vi "SpectrometerSpinCoater_v09.vi"() -> ()   [LabVIEW 2018]
uses:
  <instrlib>/Classes/CCD/Abstract_CCD/Abstract_CCD.lvclass
  <instrlib>/Classes/SpinCoater/SpinCoater.lvclass
  TypDef/DeviceQueue_TypeDef.ctl
  TypDef/DeviceQueue_Action.ctl
  TypDef/TabControl.ctl
  TypDef/DataQueue_TypeDef.ctl
  TypDef/DataQueue_Action.ctl
  <vilib>/Utility/error.llb/DialogType.ctl
  <instrlib>/Classes/CCD/Avantes/Avantes.lvclass
  C:/Program Files/National Instruments/LabVIEW 2018/instr.lib/Classes/CCD/Abstract_CCD/Abstract_CCD.lvclass
  <vilib>/Analysis/baseanly.llb/A x Vector.vi
  <vilib>/Analysis/NI_AALBase.lvlib
panel:
  out "Nr After Spin":u16
  out "Action":string="TimeOut"
  out "Time.spin":refnum<file>
  out "Meas.spin":refnum<file>
  out "Arduino":bool
  out "NKT":bool
  out "Spectromter":bool
  in  "Abort Button":bool
  in  "Stop Button":bool=TRUE
  in  "Tab Control":T1(tab)=enum."Settings"
  in  "Spin at end":bool
  in  "Duration after":dbl[unit]
  in  "periodic time":dbl[unit]
  in  "Program Spin Coater":T2(array[cluster])=[{"Speed (rpm)"=800.0, "Time (s)"=120.0, "Acc (rpm/s)"=0.0}]
  in  "Spectra Count":u16
  in  "Measure_MeasureSpectrum":bool
  out "Overall Time":dbl=121.5
  in  "Seconds after Spin":dbl[unit]=0.5
  in  "Seconds to Spin":dbl[unit]=1.0
  in  "Calculate Frames":bool=TRUE
  in  "Frames":i32=319737
  in  "StartMeasurement_Button":bool
  in  "Measure_Preview":bool
  out "Measure_Graph":T3(graph) caption="XY Graph"
  in  "Measure_FramesSpectrometer":dbl=200.0 caption="Frames for Spectrometer"
  in  "StartSpin_Button":bool
  in  "Record RefSpec":bool
  in  "Measure:\nRecord_Darkspec":bool
  in  "Measure_Comments":string="TL,  60°C, Blend P3HT 30g/L Verhältnis 1:1,2 PC70BM 24 g/L\nAuftrag während dem Spin\n" caption="Comments"
  in  "Measure_FileName":string="190624_JZ_P3HTPC70BM_TL_G17" caption="File Name"
  in  "Measure_SavePath":path=path "C:/Users/Cerberus/Desktop/Measurements" caption="Save Path"
  out "Measure_FrameRate":dbl[unit]=2631.5791015625 caption="Frame Rate"
  in  "Measure_IntegrationTime":dbl[unit]=3e-05 caption="Integration Time"
  out "SS_StepsLeft":dbl
  out "SS_TimePrediction":dbl[unit]
  out "Horizontal Progress Bar":u8(slide) scale=0.0..100.0
  in  "SpectralStability:\nRecord_Darkspec":bool
  in  "SpectralStability_Record":bool
  in  "SpectralStability_\nMeasurementNumber":u32 caption="Measurement Number"
  in  "SpectralStability_Duration":dbl[unit] caption="Duration"
  in  "Duration/Times":bool
  in  "SpectralStability_\nPeriodicTime":dbl[unit] caption="Periodic Time"
  in  "SpectralStability_MeasureSpectrum":bool
  in  "SpectralStability_Preview":bool
  out "SpectralStability_Graph":T3(graph) caption="XY Graph"
  in  "SpectralStability_FramesSpectrometer":dbl=200.0 caption="Frames for Spectrometer"
  in  "SpectralStability_Comments":string="Just for testing" caption="Comments"
  in  "SpectralStability_FileName":string="TestingAfter" caption="File Name"
  in  "SpectralStability_SavePath":path=path "C:/Users/Timo/Desktop/Test/180824" caption="Save Path"
  out "SpectralStability_FrameRate":dbl[unit]=2631.5791015625 caption="Frame Rate"
  in  "SpectralStability_IntegrationTime":dbl[unit]=3e-05 caption="Integration Time"
  in  "Dividider Get Spectra":u32=1 min=1
  in  "Automatically \nadjust count":bool=TRUE
  in  "Reset Count\nafter Spin Coating":bool=TRUE
  in  "Speed":dbl
  in  "Milliseconds":dbl
  in  "Debug":bool
  in  "Port Arduino":refnum<visa-resource-name>="COM7"
  out "Error Arduino":bool caption="Error"
  in  "Init_Arduino":bool caption="Init"
  out "Caption_Settings_Arduino":string="Arduino"
  out "Caption_Settings_NKT":string="NKT Laser"
  out "Error_Spectromter":bool caption="Error"
  in  "Init_Spectrometer":bool caption="Init"
  out "Caption_Settings_Spectrometer":string="Spectromter"
  # "Speed (rpm)   Time (s)        Acceleration \n                                               (rpm/s)"
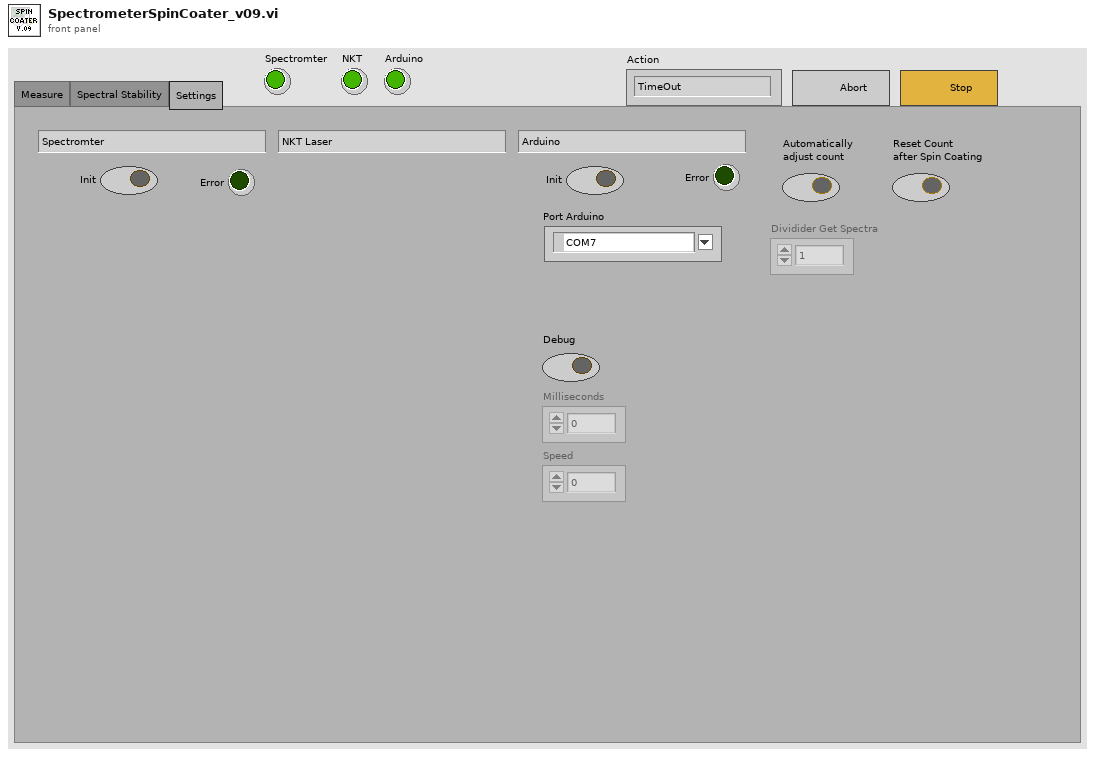
[diagram p1: front panel]
types:
  T1 = enum32{"Measure", "Spectral Stability", "Settings"}
  T2 = cluster{"Speed (rpm)":dbl, "Time (s)":dbl, "Acc (rpm/s)":dbl}[]
  T3 = cluster{"Wavlength":dbl[unit][], "Image":dbl[]}[]
  T4 = cluster{"Dark":cluster{"Image":dbl[][][], "Frame Size":cluster{"F":i32, "Y":i32, "X":i32}}[], "Ref":cluster{"Image":dbl[][][], "Frame Size":cluster{"F":i32, "Y":i32, "X":i32}}[], "Wavlength":dbl[unit][], "spec":dbl[][]}
  T5 = cluster{"Abstract_CCD.lvclass":refnum<class "Abstract_CCD.lvclass">, "SpinCoater.lvclass":refnum<class "SpinCoater.lvclass">}
  T6 = typedef "DataQueue_TypeDef.ctl" = cluster{"QueueAction":T7, "Data":cluster{"Image":dbl[][][], "Frame Size":cluster{"F":i32, "Y":i32, "X":i32}}[], "Data_Raw":cluster{"Image":dbl[][][], "Frame Size":cluster{"F":i32, "Y":i32, "X":i32}}[], "Data_Dark":cluster{"Image":dbl[][][], "Frame Size":cluster{"F":i32, "Y":i32, "X":i32}}[], "Data_Ref":cluster{"Image":dbl[][][], "Frame Size":cluster{"F":i32, "Y":i32, "X":i32}}[], "Device Information":string[], "Numeric Control":dbl, "Boolean":bool, "Wavelength":dbl[unit][], "Time":dbl[], "Time Stamp":timestamp, "Numeric Control 2":dbl, "TabControl":T8}
  T7 = typedef "DataQueue_Action.ctl" = enum16{"TimeOut", "Close_Program", "Abort", "Stop_Measurement", "Measure_InSituSpinCoating", "Measure_Spectrum", "Measure_SpectrumAdvanced", "Measure_SpectralStability", "Save_InSitu", "Save_SpectralStability", "Set_Ref", "Set_Dark", "Set_Wavelength", "Spectrometer_Measure", "Spectrometer_Preview", "Transfer_Settings"}
  T8 = typedef "TabControl.ctl" = enum16{"Measure", "Spectral Stability", "Settings"}
  T9 = typedef "DeviceQueue_TypeDef.ctl" = cluster{"QueueAction":T10, "Numeric 1":dbl, "Numeric 2":dbl, "Boolean 1":bool, "Boolean 2":bool, "Spin Program":dbl[][], "Spin Prg v07":cluster{"Speed (rpm)":dbl, "Time (s)":dbl, "Acc (rpm/s)":dbl}[], "Time Stamp":timestamp, "TabControl":T8}
  T10 = typedef "DeviceQueue_Action.ctl" = enum16{"TimeOut", "Wait", "Close_Program", "Abort", "Spectrometer_Init", "Spectrometer_Close", "Spectrometer_DeviceInformation", "Spectrometer_Measure", "Spectrometer_MeasureAdvanced", "Spectrometer_Preview", "Spectrometer_Abort", "Spectrometer_StartMeasurement", "Spectrometer_GetData", "Spectrometer_StopMeasurement", "Spectrometer_SetIntegrationTime", "Spectrometer_SetFrames", "Spectrometer_SetDarkspec", "Spectrometer_SetReference", "Spectrometer_SetTriggerMode", "Laser_Init", "Laser_Close", "Arduino_Init", "Arduino_Close", "Arduino_LoadProgram", "Arduino_StartProgram", "Arduino_SetSpeed", "Arduino_SetMillis", "Arduino_StopSpin", "Measure_InSitu", "Measure_Spectrum", "Measure_InSituAdvanced", "Measure_SpectralStability", "Measure_Stop"}
  T11 = cluster{"Image":dbl[][][], "Frame Size":cluster{"F":i32, "Y":i32, "X":i32}}[]
  T12 = typedef "DialogType.ctl" = u16
  T13 = enum16{"open", "replace", "create", "open or create", "replace or create", "replace or create with confirmation"}
  T14 = cluster{"Image":dbl[][][], "Frame Size":cluster{"F":i32, "Y":i32, "X":i32}}
  T15 = cluster{"Wavlength":dbl[unit][], "A x Vector":dbl[]}
  T16 = cluster{"Wavlength":dbl[unit][], "A x Vector":dbl[]}[]
  T17 = cluster{u16[][][], u16[][][], dbl[], "Numeric Control":dbl, "Numeric Control 2":dbl}
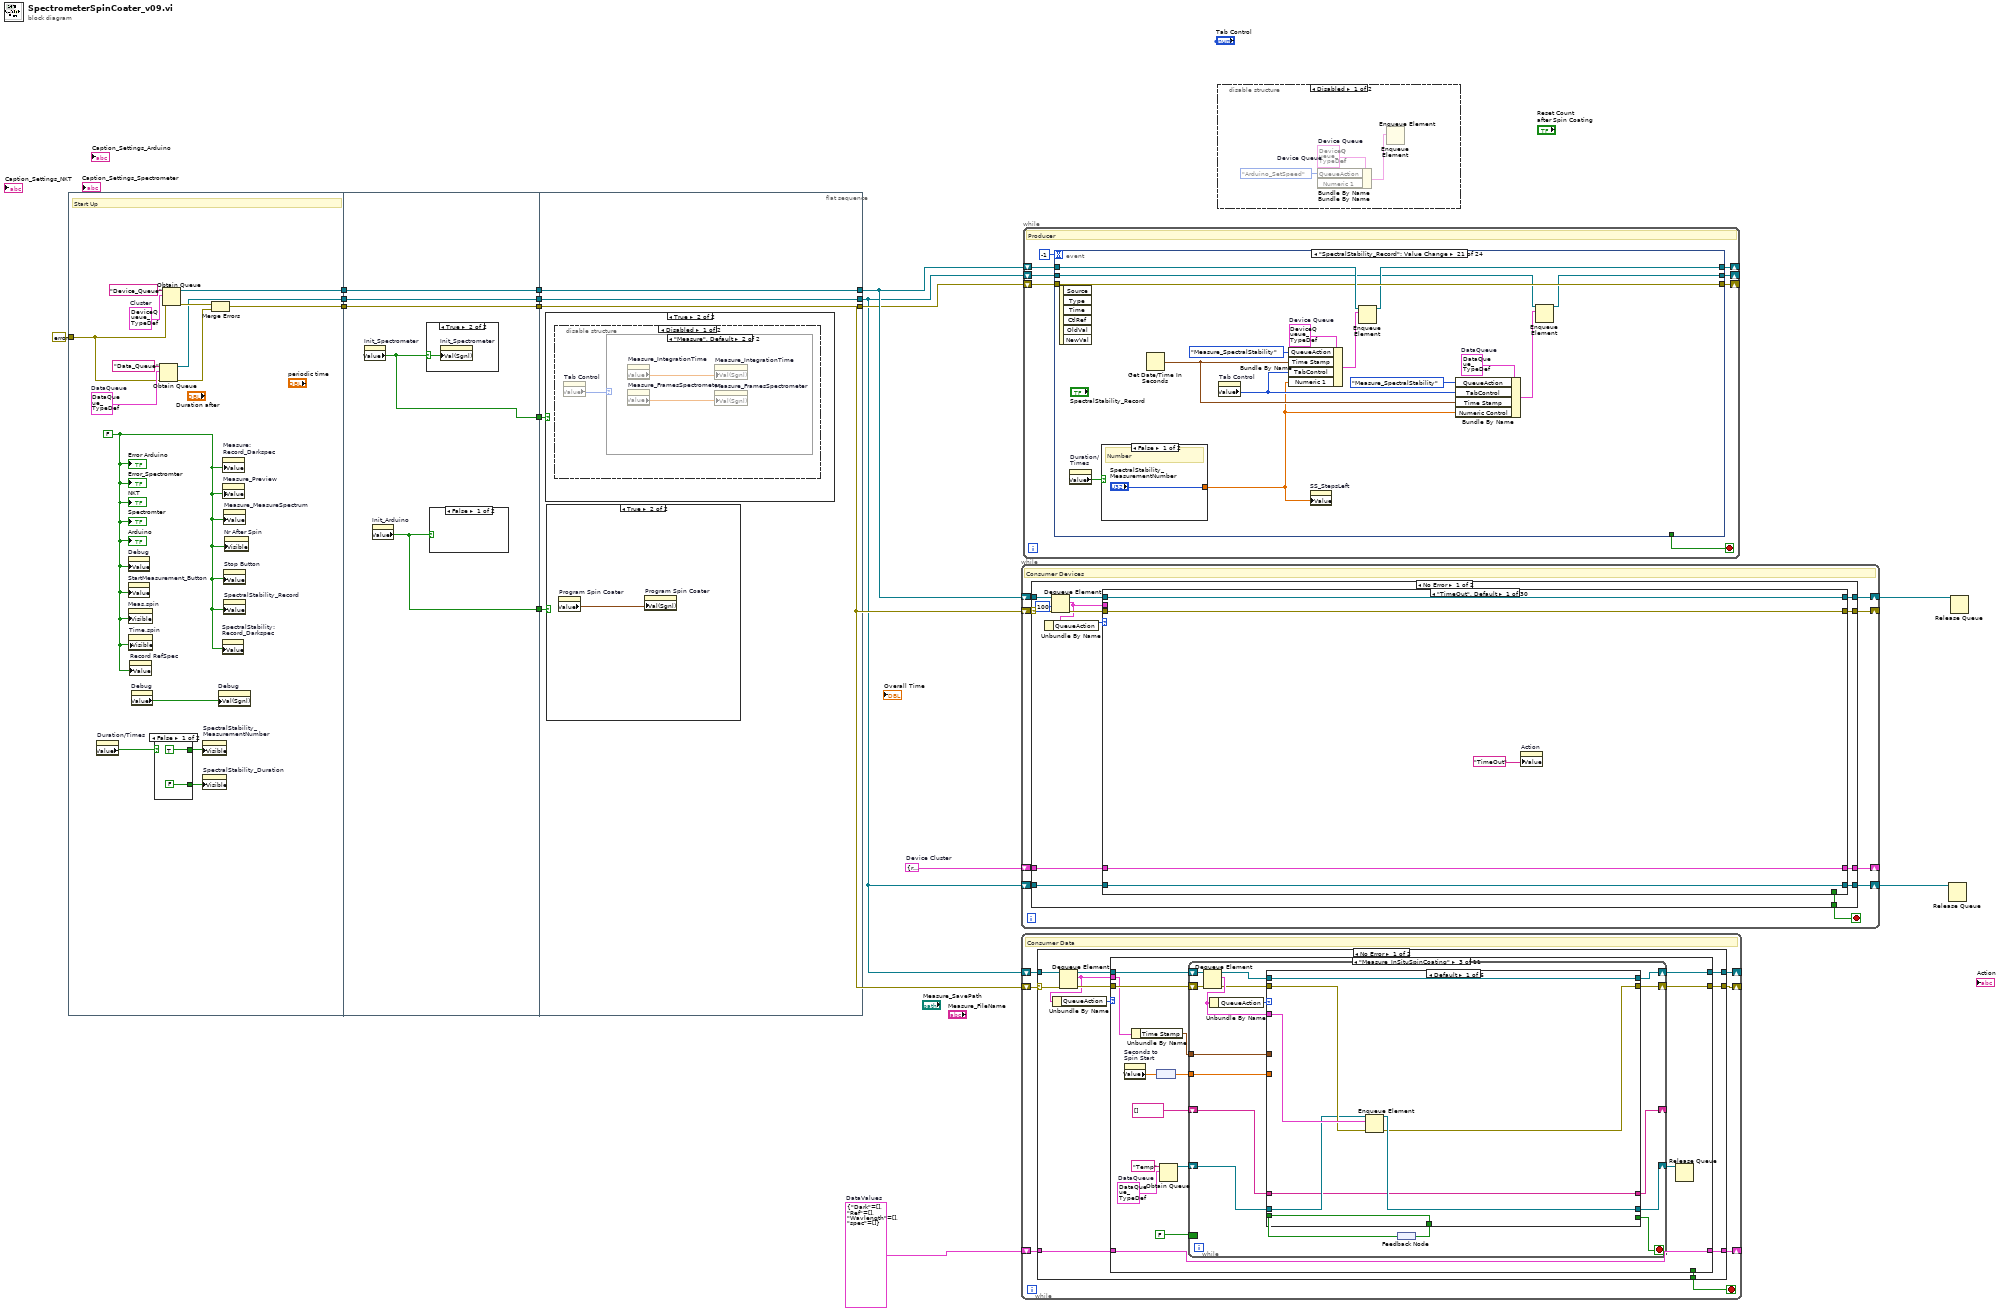
[diagram p0: block diagram]
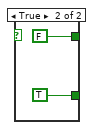
[diagram p3: hidden frame]
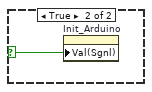
[diagram p4: hidden frame]
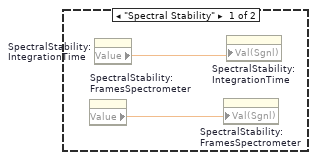
[diagram p8: hidden frame]
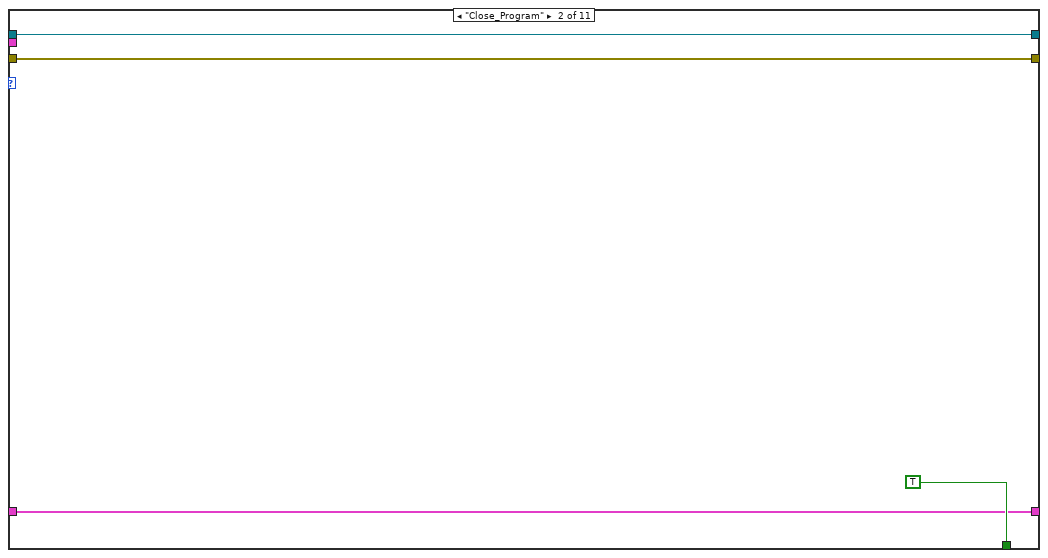
[diagram p11: hidden frame]
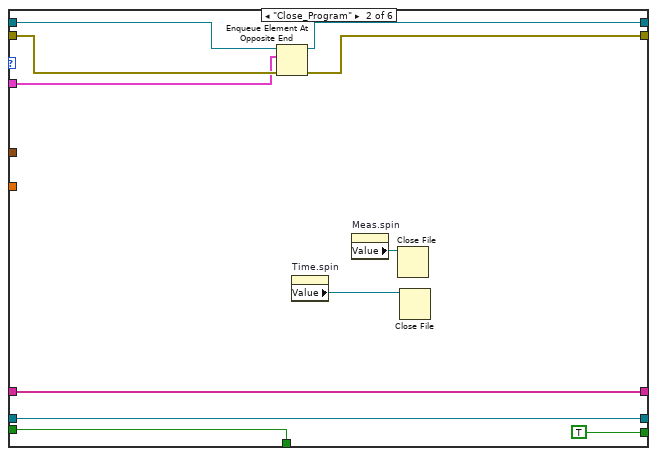
[diagram p12: hidden frame]
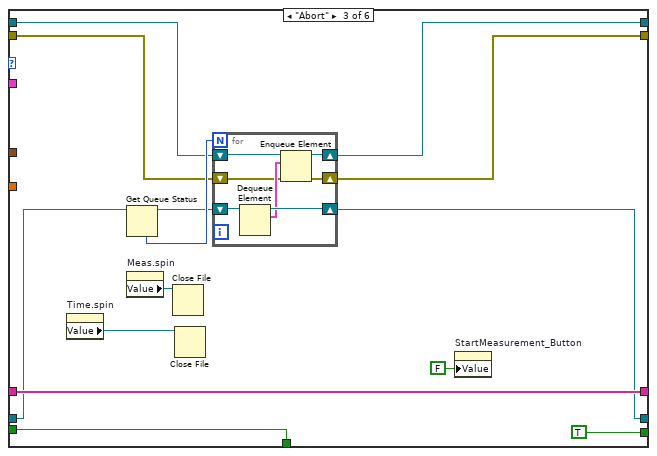
[diagram p13: hidden frame]
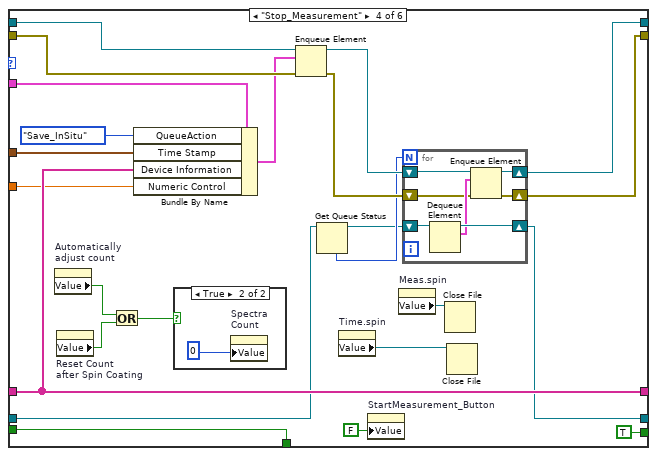
[diagram p14: hidden frame]
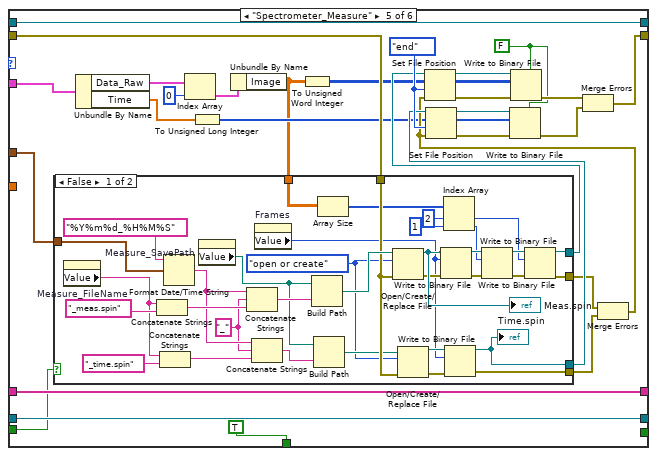
[diagram p16: hidden frame]
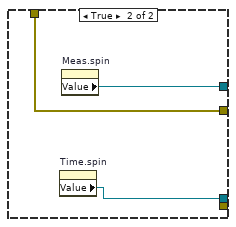
[diagram p17: hidden frame]
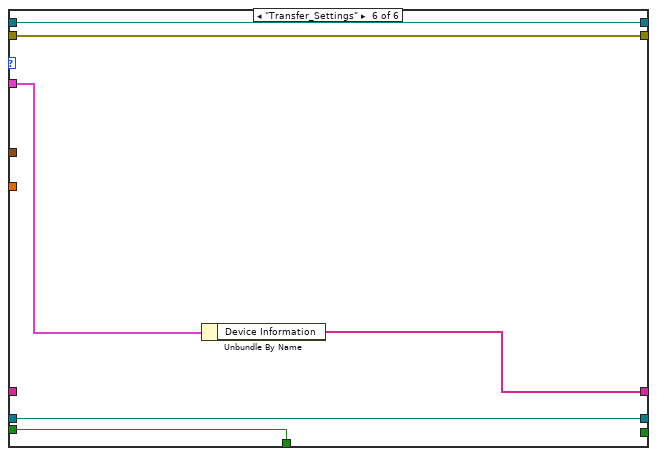
[diagram p18: hidden frame]
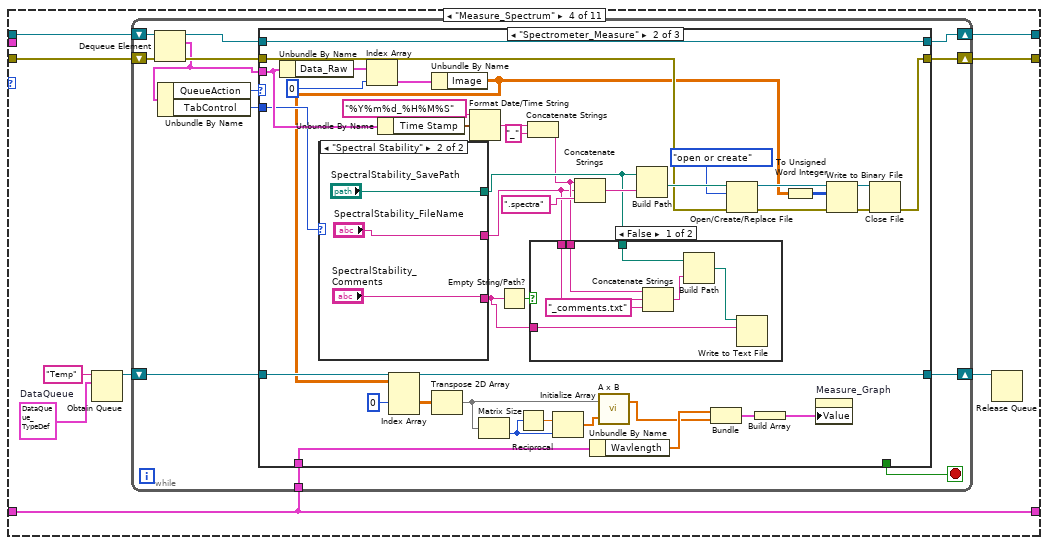
[diagram p19: hidden frame]
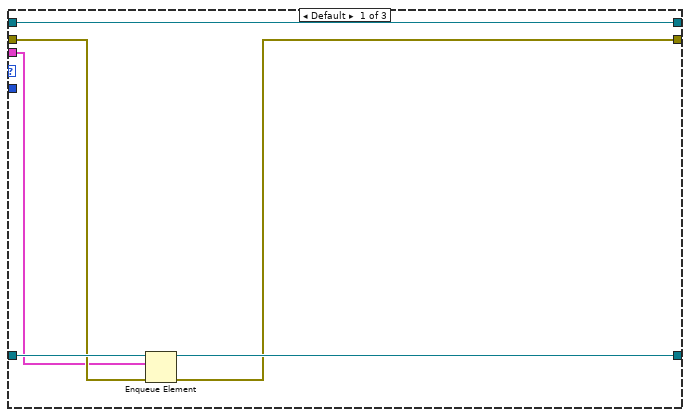
[diagram p20: hidden frame]
diagram:
  w6 = T4 {"Dark"=[], "Ref"=[], "Wavlength"=[], "spec"=[]}  # DataValues
  w11 = T5 {"Abstract_CCD.lvclass"=refnum, "SpinCoater.lvclass"=refnum}  # Device Cluster
  n1 = flat-sequence {
    tunnel: errorcluster {"status"=FALSE, "code"=0, "source"=""} ("error constant") -> [w26]
    tunnel: [w29] -> w15
    tunnel: [w23] -> w14
    tunnel: [w22] -> w13
    tunnel: w15 -> [w40]
    tunnel: w14 -> [w39]
    tunnel: w13 -> [w38]
    tunnel: [w40] -> w5
    tunnel: [w39] -> w4
    tunnel: [w38] -> w3
    tunnel: [w37] -> w2
    tunnel: [w36] -> w1
    tunnel: [w45] -> w8
    tunnel: [w46] -> w7
    tunnel: [w47] -> w12
    tunnel: w5 -> [w47]
    tunnel: w4 -> [w46]
    tunnel: w3 -> [w45]
    tunnel: w2 -> [w44]
    tunnel: w1 -> [w43]
    frame #0 {
      w27 = T6 {"QueueAction"=enum."TimeOut", "Data"=[], "Data_Raw"=[], "Data_Dark"=[], "Data_Ref"=[], "Device Information"=[], "Numeric Control"=0.0, "Boolean"=FALSE, "Wavelength"=[], "Time"=[], "Time Stamp"=timestamp(0 s since 1904-01-01), "Numeric Control 2"=0.0, "TabControl"=enum."Measure"}  # DataQueue
      w30 = T9 {"QueueAction"=enum."TimeOut", "Numeric 1"=0.0, "Numeric 2"=0.0, "Boolean 1"=FALSE, "Boolean 2"=FALSE, "Spin Program"=[], "Spin Prg v07"=[], "Time Stamp"=timestamp(0 s since 1904-01-01), "TabControl"=enum."Measure"}  # Cluster
      w17 = FALSE ("Error Arduino")
      # "Start Up"
      n2 = property on="Duration/Times" class="Bool (strict)"() -> ("Value"=w18:bool)  [unwired: 2 in, 2 out]
      n3 = property on="Debug" class="Bool (strict)"("Value"=w17) -> ()  [unwired: 2 in, 2 out]
      n4 = property on="StartMeasurement_Button" class="Bool (strict)"("Value"=w17) -> ()  [unwired: 2 in, 2 out]
      n5 = property on="Meas.spin" class="Ref (strict)"("Visible"=w17) -> ()  [unwired: 2 in, 2 out]
      n6 = property on="Time.spin" class="Ref (strict)"("Visible"=w17) -> ()  [unwired: 2 in, 2 out]
      n7 = property on="Record RefSpec" class="Bool (strict)"("Value"=w17) -> ()  [unwired: 2 in, 2 out]
      n8 = property on="Debug" class="Bool (strict)"() -> ("Value"=w21:bool)  [unwired: 2 in, 2 out]
      n9 = case shown="False" w18 {
        tunnel: [FALSE TRUE] -> w20
        tunnel: [TRUE FALSE] -> w19
        frame False {
        }
        frame True {
        }
      }
      n10 = Obtain Queue(name (unnamed)="Data_Queue", element data type=w27, error in (no error)=w26) -> (queue out=w23:refnum<queue>, error out=w24:errorcluster)  [unwired: 2 in, 1 out]
      n11 = Obtain Queue(name (unnamed)="Device_Queue", element data type=w30, error in (no error)=w26) -> (queue out=w29:refnum<queue>, error out=w25:errorcluster)  [unwired: 2 in, 1 out]
      n12 = property on="SpectralStability_\nMeasurementNumber" class="DigNum (strict)"("Visible"=w19) -> ()  [unwired: 2 in, 2 out]
      n13 = property on="SpectralStability_Duration" class="DigNum (strict)"("Visible"=w20) -> ()  [unwired: 2 in, 2 out]
      n14 = Merge Errors(w25, w24) -> (w22:errorcluster)
      n15 = property on="Debug" class="Bool (strict)"("Val(Sgnl)"=w21) -> ()  [unwired: 2 in, 2 out]
      n16 = property on="SpectralStability:\nRecord_Darkspec" class="Bool (strict)"("Value"=w17) -> ()  [unwired: 2 in, 2 out]
      n17 = property on="Measure:\nRecord_Darkspec" class="Bool (strict)"("Value"=w17) -> ()  [unwired: 2 in, 2 out]
      n18 = property on="Measure_Preview" class="Bool (strict)"("Value"=w17) -> ()  [unwired: 2 in, 2 out]
      n19 = property on="Measure_MeasureSpectrum" class="Bool (strict)"("Value"=w17) -> ()  [unwired: 2 in, 2 out]
      n20 = property on="Stop Button" class="Bool (strict)"("Value"=w17) -> ()  [unwired: 2 in, 2 out]
      n21 = property on="SpectralStability_Record" class="Bool (strict)"("Value"=w17) -> ()  [unwired: 2 in, 2 out]
      n22 = property on="Nr After Spin" class="DigNum (strict)"("Visible"=w17) -> ()  [unwired: 2 in, 2 out]
      "Error_Spectromter" <- w17
      "Error Arduino" <- w17
      "Spectromter" <- w17
      "NKT" <- w17
      "Arduino" <- w17
    }
    frame #1 {
      n23 = property on="Init_Spectrometer" class="Bool (strict)"() -> ("Value"=w37:bool)  [unwired: 2 in, 2 out]
      n24 = property on="Init_Arduino" class="Bool (strict)"() -> ("Value"=w36:bool)  [unwired: 2 in, 2 out]
      n25 = case shown="True" w37 {
        selector: w37 -> [_ w42]
        frame False {
        }
        frame True {
          n26 = property on="Init_Spectrometer" class="Bool (strict)"("Val(Sgnl)"=w42) -> ()  [unwired: 2 in, 2 out]
        }
      }
      n27 = case shown="False" w36 {
        selector: w36 -> [_ w41]
        frame False {
        }
        frame True {
          n28 = property on="Init_Arduino" class="Bool (strict)"("Val(Sgnl)"=w41) -> ()  [unwired: 2 in, 2 out]
        }
      }
    }
    frame #2 {
      n29 = case shown="True" w44 {
        frame False {
        }
        frame True {
          n30 = disable-structure shown="Disabled" {
            frame Disabled {
              n31 = property on="Tab Control" class="TabCtl (strict)"() -> ("Value"=w49:T1)  [unwired: 2 in, 2 out]
              n32 = case shown="\"Measure\", Default" w49 {
                frame "Spectral Stability" {
                  n33 = property on="SpectralStability:\nFramesSpectrometer" class="DigNum (strict)"() -> ("Value"=w50:dbl)  [unwired: 2 in, 2 out]
                  n34 = property on="SpectralStability:\nIntegrationTime" class="DigNum (strict)"() -> ("Value"=w51:dbl[unit])  [unwired: 2 in, 2 out]
                  n35 = property on="SpectralStability:\nFramesSpectrometer" class="DigNum (strict)"("Val(Sgnl)"=w50) -> ()  [unwired: 2 in, 2 out]
                  n36 = property on="SpectralStability:\nIntegrationTime" class="DigNum (strict)"("Val(Sgnl)"=w51) -> ()  [unwired: 2 in, 2 out]
                }
                frame "Measure", Default {
                  n37 = property on="Measure_IntegrationTime" class="DigNum (strict)"() -> ("Value"=w52:dbl[unit])  [unwired: 2 in, 2 out]
                  n38 = property on="Measure_FramesSpectrometer" class="DigNum (strict)"() -> ("Value"=w53:dbl)  [unwired: 2 in, 2 out]
                  n39 = property on="Measure_IntegrationTime" class="DigNum (strict)"("Val(Sgnl)"=w52) -> ()  [unwired: 2 in, 2 out]
                  n40 = property on="Measure_FramesSpectrometer" class="DigNum (strict)"("Val(Sgnl)"=w53) -> ()  [unwired: 2 in, 2 out]
                }
              }
            }
            frame Enabled {
            }
          }
        }
      }
      n41 = case shown="True" w43 {
        frame False {
        }
        frame True {
          n42 = property on="Program Spin Coater" class="Arr (strict)"() -> ("Value"=w48:T2)  [unwired: 2 in, 2 out]
          n43 = property on="Program Spin Coater" class="Arr (strict)"("Val(Sgnl)"=w48) -> ()  [unwired: 2 in, 2 out]
        }
      }
    }
  }
  n44 = while {
    shift-right: [w58] -> _
    shift-left: w8 -> [w62]
    shift-right: [w59] -> w10
    shift-left: w12 -> [w61]
    shift-right: [w56] -> w9
    shift-left: w7 -> [w57]
    shift-right: [w54] -> _
    shift-left: w11 -> [w55]
    stop <- w60 stop-if-true
    # "Consumer Devices"
    n45 = case shown="No Error" w62 {
      selector: w62 -> [w75 w763]
      tunnel: w61 -> [w76 w764]
      tunnel: [w72 _] -> w60
      tunnel: [w71 w764] -> w59
      tunnel: [w69 w760] -> w58
      tunnel: w57 -> [w67 w758]
      tunnel: [w68 w758] -> w56
      tunnel: w55 -> [w66 w759]
      tunnel: [w65 w759] -> w54
      frame No Error {
        n46 = Dequeue Element(queue=w76, timeout in ms (-1)=100, error in (no error)=w75) -> (queue out=w74:refnum<queue>, element=w64:T9, error out=w70:errorcluster)  [unwired: 1 out]
        n47 = Unbundle By Name(w64) -> ("QueueAction"=w73:T10)
        n48 = case shown="\"TimeOut\", Default" w73 {
          tunnel: w74 -> [w81 w102 w143 w161 w172 w227 w246 w271 w282 w305 w312 w331 w333 w364 w383 w398 w408 w420 w432 w453 w475 w480 w487 w499 w505 w515 w561 w651 w719 w729]
          tunnel: [_ _ w145 _ _ _ _ _ _ _ _ _ _ _ _ _ _ _ _ _ _ _ _ _ _ _ _ _ _ _] -> w72
          tunnel: [w81 w102 w128 w147 w168 w227 w246 w271 w283 w305 w312 w331 w333 w364 w383 w398 w408 w420 w431 w453 w475 w480 w487 w499 w505 w515 w523 w577 w710 w732] -> w71
          tunnel: w70 -> [w80 w101 w127 w160 w183 w228 w245 w270 w278 w308 w316 w328 w343 w362 w373 w389 w405 w416 w427 w456 w469 w477 w485 w494 w502 w508 w517 w612 w718 w728]
          tunnel: [w80 w101 w126 w148 w171 w222 w244 w269 w276 w306 w313 w318 w337 w361 w368 w385 w403 w410 w430 w455 w466 w476 w483 w493 w501 w507 w524 w578 w709 w733] -> w69
          tunnel: [w78 w99 w125 w165 w169 w224 w237 w251 w287 w304 w311 w322 w345 w365 w377 w392 w399 w412 w434 w454 w474 w482 w491 w497 w506 w510 w532 w624 w717 w749] -> w68
          tunnel: w67 -> [w78 w99 w125 w165 w170 w224 w236 w260 w288 w304 w311 w323 w345 w365 w380 w395 w399 w414 w434 w454 w474 w482 w491 w497 w506 w511 w532 w624 w717 w749]
          tunnel: w66 -> [w79 w100 w124 w164 w180 w226 w243 w268 w281 w303 w315 w324 w336 w358 w376 w391 w402 w409 w429 w449 w468 w481 w490 w496 w504 w509 w564 w654 w716 w748]
          tunnel: [w79 w100 w124 w164 w174 w225 w243 w268 w280 w301 w310 w324 w334 w359 w375 w390 w400 w409 w433 w447 w465 w481 w490 w496 w504 w509 w564 w654 w716 w748] -> w65
          tunnel: w64 -> [_ w95 _ _ w167 _ w235 w262 w274 _ _ w330 w340 w366 _ _ w406 _ _ _ w473 _ w489 w498 _ _ _ w594 w707 w723]
          frame "TimeOut", Default {
            n49 = property on="Action" class="Str"("Value"="TimeOut" ("Action")) -> ()  [unwired: 2 in, 2 out]
          }
          frame "Wait" {
            n50 = flat-sequence {
              tunnel: [w113] -> w96
              tunnel: w95 -> [w113]
              tunnel: [w112] -> w93
              frame #0 {
                n51 = Tick Count (ms)() -> (millisecond timer value=w112:u32)
              }
            }
            n52 = Unbundle By Name(w96) -> ("Numeric 1"=w87:dbl)
            n53 = property on="SS:PeriodicTime" class="DigNum (strict)"() -> ("Value"=w89:dbl[unit])  [unwired: 2 in, 2 out]
            n54 = Multiply(x=w87, y=1000.0) -> (x*y=w91:dbl)
            n55 = node(w87) -> (w88:dbl[unit])
            n56 = property on="SS_StepsLeft" class="DigNum (strict)"() -> ("Value"=w86:dbl)  [unwired: 2 in, 2 out]
            n57 = Round Toward -Infinity(1:w87) -> (0:w90:dbl)
            n58 = Subtract(x=w89, y=w88) -> (x-y=w83:dbl[unit])
            n59 = Decrement(x=w86) -> (x-1=w85:dbl)
            n60 = Multiply(x=w85, y=w89) -> (x*y=w84:dbl[unit])
            n61 = Add(x=w84, y=w83) -> (x+y=w82:dbl[unit])
            n62 = for {
              N: w90 -> [_]
              tunnel: 1000.0 ("y") -> [w114]
              tunnel: [w122] -> w94
              tunnel: w82 -> [w119]
              i -> [w117]
              stop <- w122 stop-if-true
              n63 = Increment(x=w117) -> (x+1=w115:i32)
              n64 = Multiply(x=w114, y=w115) -> (x*y=w116:dbl)
              n65 = node(w116) -> (w118:dbl[unit])
              n66 = property on="Stop Button" class="Bool (strict)"() -> ("Value"=w122:bool)  [unwired: 2 in, 2 out]
              n67 = Wait (ms)(milliseconds to wait=w114) -> (millisecond timer value=w120:u32)
              n68 = Subtract(x=w119, y=w118) -> (x-y=w121:dbl[unit])
              n69 = flat-sequence {
                tunnel: w121 -> [w123]
                tunnel: w120 -> [_]
                frame #0 {
                  n70 = property on="SS_TimePrediction" class="DigNum (strict)"("Value"=w123) -> ()  [unwired: 2 in, 2 out]
                }
              }
            }
            n71 = property on="Action" class="Str"("Value"="Wait" ("Action")) -> ()  [unwired: 2 in, 2 out]
            n72 = case shown="False" w94 {
              tunnel: w93 -> [w108 _]
              tunnel: w91 -> [w103 _]
              frame False {
                n73 = flat-sequence {
                  tunnel: [w111] -> w109
                  frame #0 {
                    n74 = Tick Count (ms)() -> (millisecond timer value=w111:u32)
                  }
                }
                n75 = Subtract(x=w109, y=w108) -> (x-y=w107:u32)
                n76 = To Double Precision Float(number=w107) -> (double precision float=w104:dbl)
                n77 = Subtract(x=w103, y=w104) -> (x-y=w105:dbl)
                n78 = Greater Than 0?(x=w105) -> (x > 0?=w106:bool)
                n79 = case shown="True" w106 {
                  tunnel: w105 -> [_ w110]
                  frame False {
                  }
                  frame True {
                    n80 = Wait (ms)(milliseconds to wait=w110) -> ()  [unwired: 1 out]
                  }
                }
              }
              frame True {
                # "If Aborted, do nothing"
              }
            }
          }
          frame "Close_Program" {
            w144 = T9 {"QueueAction"=enum."TimeOut", "Numeric 1"=0.0, "Numeric 2"=0.0, "Boolean 1"=FALSE, "Boolean 2"=FALSE, "Spin Program"=[], "Spin Prg v07"=[], "Time Stamp"=timestamp(0 s since 1904-01-01), "TabControl"=enum."Measure"}  # Device Queue
            n81 = Bundle By Name(cluster=w144, "QueueAction"=DeviceQueue_Action."Spectrometer_Close") -> (w139:T9)
            n82 = Bundle By Name(cluster=w139, "QueueAction"=DeviceQueue_Action."Laser_Close") -> (w137:T9)
            n83 = Bundle By Name(cluster=w137, "QueueAction"=DeviceQueue_Action."Arduino_Close") -> (w131:T9)
            n84 = Enqueue Element(queue=w143, element=w139, error in (no error)=w127) -> (queue out=w141:refnum<queue>, error out=w136:errorcluster)  [unwired: 1 in, 1 out]
            n85 = Bundle By Name(cluster=w131, "QueueAction"=DeviceQueue_Action."Close_Program") -> (w129:T9)
            n86 = Enqueue Element(queue=w141, element=w137, error in (no error)=w136) -> (queue out=w135:refnum<queue>, error out=w134:errorcluster)  [unwired: 1 in, 1 out]
            n87 = Enqueue Element(queue=w135, element=w131, error in (no error)=w134) -> (queue out=w133:refnum<queue>, error out=w132:errorcluster)  [unwired: 1 in, 1 out]
            n88 = Enqueue Element(queue=w133, element=w129, error in (no error)=w132) -> (queue out=w128:refnum<queue>, error out=w126:errorcluster)  [unwired: 1 in, 1 out]
            n89 = First Call?() -> (First Call?: T/F=w146:bool)
            n90 = Not(x=w146) -> (.not. x?=w145:bool)
          }
          frame "Abort" {
            w163 = T9 {"QueueAction"=enum."TimeOut", "Numeric 1"=0.0, "Numeric 2"=0.0, "Boolean 1"=FALSE, "Boolean 2"=FALSE, "Spin Program"=[], "Spin Prg v07"=[], "Time Stamp"=timestamp(0 s since 1904-01-01), "TabControl"=enum."Measure"}  # Device Queue
            n91 = Flush Queue(queue=w161, error in (no error)=w160) -> (queue out=w159:refnum<queue>, error out=w158:errorcluster)  [unwired: 1 out]
            n92 = Bundle By Name(cluster=w163, "QueueAction"=DeviceQueue_Action."Spectrometer_StopMeasurement") -> (w155:T9)
            n93 = Bundle By Name(cluster=w155, "QueueAction"=DeviceQueue_Action."Arduino_StopSpin") -> (w151:T9)
            n94 = Enqueue Element(queue=w159, element=w155, error in (no error)=w158) -> (queue out=w157:refnum<queue>, error out=w156:errorcluster)  [unwired: 1 in, 1 out]
            n95 = Bundle By Name(cluster=w151, "QueueAction"=DeviceQueue_Action."Measure_Stop") -> (w150:T9)
            n96 = Enqueue Element(queue=w157, element=w151, error in (no error)=w156) -> (queue out=w153:refnum<queue>, error out=w152:errorcluster)  [unwired: 1 in, 1 out]
            n97 = Enqueue Element(queue=w153, element=w150, error in (no error)=w152) -> (queue out=w147:refnum<queue>, error out=w148:errorcluster)  [unwired: 1 in, 1 out]
          }
          frame "Spectrometer_Init" {
            n98 = call-dynamic "Init.vi"("error in (no error)"=w183, "Variant"=0, "Avantes in"=refnum<class "Avantes.lvclass"> refnum ("Avantes.lvclass")) -> ("error out"=w182:errorcluster, "Avantes out"=w181:refnum<class "Avantes.lvclass">)  [unwired: 7 in]
            n99 = call-dynamic "IsInit.vi"("error in (no error)"=w182, "Avantes in"=w181) -> ("error out"=w178:errorcluster, "Is Init?"=w177:bool, "Avantes out"=w179:refnum<class "Avantes.lvclass">)  [unwired: 7 in]
            n100 = Unbundle By Name(w167) -> ("TabControl"=w166:T8)
            n101 = property on="Spectromter" class="Bool (strict)"("Value"=w177) -> ()  [unwired: 2 in, 2 out]
            n102 = property on="Init_Spectrometer" class="Bool (strict)"("Value"=w177) -> ()  [unwired: 2 in, 2 out]
            n103 = call-dynamic "Set_ExposurePerFrame.vi"("error in (no error)"=w178, "Exposure per Frame"=1, "Avantes in"=w179) -> ("error out"=w173:errorcluster, "Avantes out"=w176:refnum<class "Avantes.lvclass">)  [unwired: 7 in]
            n104 = case shown="False" w177 {
              tunnel: w176 -> [_ w206]
              tunnel: w173 -> [w189 w204]
              tunnel: [refnum<class "Abstract_CCD.lvclass"> refnum ("Abstract_CCD.lvclass") w205] -> w175
              tunnel: w172 -> [w187 w216]
              tunnel: [w189 w209] -> w171
              tunnel: w170 -> [w188 w201]
              tunnel: [w188 w199] -> w169
              tunnel: [w187 w197] -> w168
              tunnel: w167 -> [_ w194]
              tunnel: w166 -> [_ w193]
              frame False {
              }
              frame True {
                w207 = T6 {"QueueAction"=enum."TimeOut", "Data"=[], "Data_Raw"=[], "Data_Dark"=[], "Data_Ref"=[], "Device Information"=[], "Numeric Control"=0.0, "Boolean"=FALSE, "Wavelength"=[], "Time"=[], "Time Stamp"=timestamp(0 s since 1904-01-01), "Numeric Control 2"=0.0, "TabControl"=enum."Measure"}  # DataQueue
                n105 = case shown="\"Spectral Stability\"" w193 {
                  tunnel: [w218 w220] -> w192
                  tunnel: [w217 w219] -> w191
                  frame "Measure", Default {
                    n106 = property on="Measure_IntegrationTime" class="DigNum (strict)"() -> ("Value"=w218:dbl[unit])  [unwired: 2 in, 2 out]
                    n107 = property on="Measure_FramesSpectrometer" class="DigNum (strict)"() -> ("Value"=w217:dbl)  [unwired: 2 in, 2 out]
                  }
                  frame "Spectral Stability" {
                    n108 = property on="SpectralStability_FramesSpectrometer" class="DigNum (strict)"() -> ("Value"=w219:dbl)  [unwired: 2 in, 2 out]
                    n109 = property on="SpectralStability_IntegrationTime" class="DigNum (strict)"() -> ("Value"=w220:dbl[unit])  [unwired: 2 in, 2 out]
                  }
                }
                n110 = call-dynamic "Get_WavelengthAxis.vi"("error in (no error)"=w204, "Avantes in"=w206) -> ("error out"=w203:errorcluster, "lambda"=w198:dbl[unit][], "Avantes out"=w205:refnum<class "Avantes.lvclass">)  [unwired: 7 in]
                n111 = Unbundle(w203) -> ("status"=w202:bool)  [unwired: 2 out]
                n112 = property on="Error_Spectromter" class="Bool (strict)"("Value"=w202) -> ()  [unwired: 2 in, 2 out]
                n113 = property on="Calculate Frames" class="Bool (strict)"() -> ("Value"=w195:bool)  [unwired: 2 in, 2 out]
                n114 = Bundle By Name(cluster=w207, "QueueAction"=DataQueue_Action."Set_Wavelength", "Wavelength"=w198) -> (w208:T6)
                n115 = node(w192) -> (w214:dbl)
                n116 = Bundle By Name(cluster=w194, "QueueAction"=DeviceQueue_Action."Spectrometer_SetIntegrationTime", "Numeric 1"=w214, "Boolean 1"=w195) -> (w212:T9)
                n117 = Enqueue Element(queue=w201, element=w208) -> (queue out=w199:refnum<queue>)  [unwired: 2 in, 2 out]
                n118 = Bundle By Name(cluster=w212, "QueueAction"=DeviceQueue_Action."Spectrometer_SetFrames", "Numeric 1"=w191) -> (w211:T9)
                n119 = Enqueue Element(queue=w216, element=w212, error in (no error)=w204) -> (queue out=w213:refnum<queue>, error out=w210:errorcluster)  [unwired: 1 in, 1 out]
                n120 = Enqueue Element(queue=w213, element=w211, error in (no error)=w210) -> (queue out=w197:refnum<queue>, error out=w209:errorcluster)  [unwired: 1 in, 1 out]
              }
            }
            n121 = Bundle By Name(cluster=w180, "Abstract_CCD.lvclass"=w175) -> (w174:T5)
          }
          frame "Spectrometer_Close" {
            n122 = property on="Spectromter" class="Bool (strict)"("Value"=FALSE ("Spectromter")) -> ()  [unwired: 2 in, 2 out]
            n123 = Unbundle By Name(w226) -> ("Abstract_CCD.lvclass"=w229:refnum<class "Abstract_CCD.lvclass">)
            n124 = flat-sequence {
              tunnel: [refnum<class "Abstract_CCD.lvclass"> refnum ("Abstract_CCD.lvclass")] -> w223
              tunnel: w222 -> [_]
              frame #0 {
              }
            }
            n125 = call-dynamic "Close.vi"("error in (no error)"=w228, "Abstract_CCD in"=w229) -> ("error out"=w222:errorcluster)  [unwired: 8 in, 1 out]
            n126 = Bundle By Name(cluster=w226, "Abstract_CCD.lvclass"=w223) -> (w225:T5)
          }
          frame "Spectrometer_Measure" {
            w248 = T6 {"QueueAction"=enum."TimeOut", "Data"=[], "Data_Raw"=[], "Data_Dark"=[], "Data_Ref"=[], "Device Information"=[], "Numeric Control"=0.0, "Boolean"=FALSE, "Wavelength"=[], "Time"=[], "Time Stamp"=timestamp(0 s since 1904-01-01), "Numeric Control 2"=0.0, "TabControl"=enum."Measure"}  # DataQueue
            n127 = Unbundle By Name(w243) -> ("Abstract_CCD.lvclass"=w247:refnum<class "Abstract_CCD.lvclass">)
            n128 = Unbundle By Name(w235) -> ("Time Stamp"=w232:timestamp, "TabControl"=w233:T8)
            n129 = Get Date/Time In Seconds() -> (seconds since 1Jan1904=w231:timestamp)
            n130 = Subtract(x=w231, y=w232) -> (x-y=w234:dbl)
            n131 = call-dynamic "Measure.vi"("error in (no error)"=w245, "Abstract_CCD in"=w247) -> ("error out"=w244:errorcluster, "Data Raw"=w240:T11, "Data"=w241:T11, "Darkspec"=w239:T11, "Time"=w238:dbl[])  [unwired: 3 in, 2 out]
            n132 = Bundle By Name(cluster=w248, "QueueAction"=DataQueue_Action."Spectrometer_Measure", "Data"=w241, "Data_Raw"=w240, "Data_Dark"=w239, "Time"=w238, "Time Stamp"=w232, "Numeric Control 2"=w234, "TabControl"=w233) -> (w249:T6)
            n133 = Enqueue Element(queue=w236, element=w249) -> (queue out=w237:refnum<queue>)  [unwired: 2 in, 2 out]
          }
          frame "Spectrometer_MeasureAdvanced" {
            w259 = T6 {"QueueAction"=enum."TimeOut", "Data"=[], "Data_Raw"=[], "Data_Dark"=[], "Data_Ref"=[], "Device Information"=[], "Numeric Control"=0.0, "Boolean"=FALSE, "Wavelength"=[], "Time"=[], "Time Stamp"=timestamp(0 s since 1904-01-01), "Numeric Control 2"=0.0, "TabControl"=enum."Measure"}  # DataQueue
            w273 = T6 {"QueueAction"=enum."TimeOut", "Data"=[], "Data_Raw"=[], "Data_Dark"=[], "Data_Ref"=[], "Device Information"=[], "Numeric Control"=0.0, "Boolean"=FALSE, "Wavelength"=[], "Time"=[], "Time Stamp"=timestamp(0 s since 1904-01-01), "Numeric Control 2"=0.0, "TabControl"=enum."Measure"}  # DataQueue
            n134 = Unbundle By Name(w268) -> ("Abstract_CCD.lvclass"=w272:refnum<class "Abstract_CCD.lvclass">)
            n135 = Unbundle By Name(w262) -> ("Time Stamp"=w261:timestamp)
            n136 = call-dynamic "Measure.vi"("error in (no error)"=w270, "Abstract_CCD in"=w272) -> ("error out"=w269:errorcluster, "Data Raw"=w265:T11, "Data"=w266:T11, "Darkspec"=w264:T11, "Time"=w263:dbl[])  [unwired: 3 in, 2 out]
            n137 = Bundle By Name(cluster=w259, "QueueAction"=DataQueue_Action."Measure_SpectrumAdvanced") -> (w257:T6)
            n138 = Bundle By Name(cluster=w273, "QueueAction"=DataQueue_Action."Spectrometer_Measure", "Data"=w266, "Data_Raw"=w265, "Data_Dark"=w264, "Time"=w263, "Time Stamp"=w261) -> (w254:T6)
            n139 = Enqueue Element(queue=w260, element=w257) -> (queue out=w256:refnum<queue>)  [unwired: 2 in, 2 out]
            n140 = Enqueue Element(queue=w256, element=w254) -> (queue out=w255:refnum<queue>)  [unwired: 2 in, 2 out]
            n141 = Bundle By Name(cluster=w254, "QueueAction"=DataQueue_Action."Stop_Measurement") -> (w252:T6)
            n142 = property on="Action" class="Str"("Value"="Measure Spectra A" ("Action")) -> ()  [unwired: 2 in, 2 out]
            n143 = Enqueue Element(queue=w255, element=w252) -> (queue out=w251:refnum<queue>)  [unwired: 2 in, 2 out]
          }
          frame "Spectrometer_Preview" {
            w289 = T6 {"QueueAction"=enum."TimeOut", "Data"=[], "Data_Raw"=[], "Data_Dark"=[], "Data_Ref"=[], "Device Information"=[], "Numeric Control"=0.0, "Boolean"=FALSE, "Wavelength"=[], "Time"=[], "Time Stamp"=timestamp(0 s since 1904-01-01), "Numeric Control 2"=0.0, "TabControl"=enum."Measure"}  # DataQueue
            n144 = Unbundle By Name(w281) -> ("Abstract_CCD.lvclass"=w279:refnum<class "Abstract_CCD.lvclass">)
            n145 = Unbundle By Name(w274) -> ("TabControl"=w275:T8)
            n146 = call-dynamic "Measure.vi"("error in (no error)"=w278, "Abstract_CCD in"=w279) -> ("error out"=w276:errorcluster, "Data Raw"=w286:T11, "Abstract_CCD out"=w277:refnum<class "Abstract_CCD.lvclass">)  [unwired: 3 in, 4 out]
            n147 = case shown="\"Measure\"" w275 {
              tunnel: [FALSE ("Value") w293 w294] -> w284
              tunnel: w276 -> [_ w292 _]
              frame Default {
              }
              frame "Measure" {
                n148 = property on="Measure_Preview" class="Bool (strict)"(error in=w292) -> ("Value"=w293:bool)  [unwired: 1 in, 2 out]
              }
              frame "Spectral Stability" {
                n149 = property on="SpectralStability_Preview" class="Bool (strict)"() -> ("Value"=w294:bool)  [unwired: 2 in, 2 out]
              }
            }
            n150 = case shown="True" w284 {
              tunnel: [w295 w298] -> w283
              tunnel: w282 -> [w295 w297]
              tunnel: w274 -> [_ w296]
              frame False {
              }
              frame True {
                n151 = Bundle By Name(cluster=w296, "QueueAction"=DeviceQueue_Action."Spectrometer_Preview") -> (w299:T9)
                n152 = Enqueue Element(queue=w297, element=w299) -> (queue out=w298:refnum<queue>)  [unwired: 2 in, 2 out]
              }
            }
            n153 = Bundle By Name(cluster=w289, "Data_Raw"=w286, "QueueAction"=DataQueue_Action."Spectrometer_Preview", "TabControl"=w275) -> (w290:T6)
            n154 = Enqueue Element(queue=w288, element=w290) -> (queue out=w287:refnum<queue>)  [unwired: 2 in, 2 out]
            n155 = Bundle By Name(cluster=w281, "Abstract_CCD.lvclass"=w277) -> (w280:T5)
          }
          frame "Spectrometer_StartMeasurement" {
            n156 = Unbundle By Name(w303) -> ("Abstract_CCD.lvclass"=w307:refnum<class "Abstract_CCD.lvclass">)
            n157 = call-dynamic "StartMeasure.vi"("error in (no error)"=w308, "Frames"=-1, "Abstract_CCD in"=w307) -> ("error out"=w306:errorcluster, "Abstract_CCD out"=w302:refnum<class "Abstract_CCD.lvclass">)  [unwired: 7 in]
            n158 = Bundle By Name(cluster=w303, "Abstract_CCD.lvclass"=w302) -> (w301:T5)
          }
          frame "Spectrometer_StopMeasurement" {
            n159 = Unbundle By Name(w315) -> ("Abstract_CCD.lvclass"=w317:refnum<class "Abstract_CCD.lvclass">)
            n160 = call-dynamic "StopMeasurement.vi"("error in (no error)"=w316, "Abstract_CCD in"=w317) -> ("error out"=w313:errorcluster, "Abstract_CCD out"=w314:refnum<class "Abstract_CCD.lvclass">)  [unwired: 8 in]
            n161 = Bundle By Name(cluster=w315, "Abstract_CCD.lvclass"=w314) -> (w310:T5)
          }
          frame "Spectrometer_GetData" {
            w327 = T6 {"QueueAction"=enum."TimeOut", "Data"=[], "Data_Raw"=[], "Data_Dark"=[], "Data_Ref"=[], "Device Information"=[], "Numeric Control"=0.0, "Boolean"=FALSE, "Wavelength"=[], "Time"=[], "Time Stamp"=timestamp(0 s since 1904-01-01), "Numeric Control 2"=0.0, "TabControl"=enum."Measure"}  # DataQueue
            n162 = Unbundle By Name(w324) -> ("Abstract_CCD.lvclass"=w329:refnum<class "Abstract_CCD.lvclass">)
            n163 = Unbundle By Name(w330) -> ("Numeric 1"=w321:dbl)
            n164 = call-dynamic "Measure_GetData.vi"("error in (no error)"=w328, "SpectraCount"=w321, "Abstract_CCD in"=w329) -> ("error out"=w318:errorcluster, "Data_Raw"=w320:T11, "Time"=w319:dbl[])  [unwired: 5 in, 1 out]
            n165 = Bundle By Name(cluster=w327, "QueueAction"=DataQueue_Action."Spectrometer_Measure", "Data_Raw"=w320, "Time"=w319) -> (w326:T6)
            n166 = Enqueue Element(queue=w323, element=w326) -> (queue out=w322:refnum<queue>)  [unwired: 2 in, 2 out]
          }
          frame "Spectrometer_SetIntegrationTime" {
            n167 = Unbundle By Name(w340) -> ("Numeric 1"=w342:dbl)
            n168 = Unbundle By Name(w336) -> ("Abstract_CCD.lvclass"=w344:refnum<class "Abstract_CCD.lvclass">)
            n169 = Unbundle By Name(w340) -> ("TabControl"=w332:T8, "Boolean 1"=w339:bool)
            n170 = node(w342) -> (w341:dbl[unit])
            n171 = call-dynamic "Set_ExposureTime.vi"("error in (no error)"=w343, "Exposure Time"=w341, "Abstract_CCD in"=w344) -> ("error out"=w347:errorcluster, "Abstract_CCD out"=w346:refnum<class "Abstract_CCD.lvclass">)  [unwired: 7 in]
            n172 = call-dynamic "Get_FrameRate.vi"("error in (no error)"=w347, "Abstract_CCD in"=w346) -> ("error out"=w337:errorcluster, "Frame Rate"=w338:dbl[unit], "Abstract_CCD out"=w335:refnum<class "Abstract_CCD.lvclass">)  [unwired: 7 in]
            n173 = Bundle By Name(cluster=w336, "Abstract_CCD.lvclass"=w335) -> (w334:T5)
            n174 = case shown="\"Measure\"" w332 {
              tunnel: w339 -> [_ _ w350]
              tunnel: w338 -> [_ w348 w349]
              frame Default {
              }
              frame "Spectral Stability" {
                "SpectralStability_FrameRate" <- w348
              }
              frame "Measure" {
                n175 = case shown="True" w350 {
                  tunnel: w349 -> [_ w354]
                  frame False {
                  }
                  frame True {
                    n176 = property on="Program Spin Coater" class="Arr (strict)"() -> ("Value"=w351:T2)  [unwired: 2 in, 2 out]
                    n177 = property on="Seconds to Spin" class="DigNum (strict)"() -> ("Value"=w356:dbl[unit])  [unwired: 2 in, 2 out]
                    n178 = property on="Seconds after Spin" class="DigNum (strict)"() -> ("Value"=w355:dbl[unit])  [unwired: 2 in, 2 out]
                    n179 = call "CalculateFrames_v02.vi"("Program Spin Coater"=w351, "Seconds End"=w355, "Seconds Start"=w356, "Frame Rate"=w354) -> ("Time"=w353:dbl, "Frames"=w352:i32)  [unwired: 6 in]
                    n180 = property on="Frames" class="DigNum (strict)"("Value"=w352) -> ()  [unwired: 2 in, 2 out]
                    n181 = property on="Overall Time" class="DigNum (strict)"("Value"=w353) -> ()  [unwired: 2 in, 2 out]
                  }
                }
                "Measure_FrameRate" <- w349
              }
            }
          }
          frame "Spectrometer_SetFrames" {
            n182 = Unbundle By Name(w358) -> ("Abstract_CCD.lvclass"=w363:refnum<class "Abstract_CCD.lvclass">)
            n183 = Unbundle By Name(w366) -> ("Numeric 1"=w360:dbl)
            n184 = call-dynamic "Set_Frames.vi"("error in (no error)"=w362, "Frames"=w360, "Abstract_CCD in"=w363) -> ("error out"=w361:errorcluster, "Abstract_CCD out"=w357:refnum<class "Abstract_CCD.lvclass">)  [unwired: 7 in]
            n185 = Bundle By Name(cluster=w358, "Abstract_CCD.lvclass"=w357) -> (w359:T5)
          }
          frame "Spectrometer_SetDarkspec" {
            w381 = T6 {"QueueAction"=enum."TimeOut", "Data"=[], "Data_Raw"=[], "Data_Dark"=[], "Data_Ref"=[], "Device Information"=[], "Numeric Control"=0.0, "Boolean"=FALSE, "Wavelength"=[], "Time"=[], "Time Stamp"=timestamp(0 s since 1904-01-01), "Numeric Control 2"=0.0, "TabControl"=enum."Measure"}  # DataQueue
            n186 = Unbundle By Name(w376) -> ("Abstract_CCD.lvclass"=w374:refnum<class "Abstract_CCD.lvclass">)
            n187 = call-dynamic "Measure.vi"("error in (no error)"=w373, "Abstract_CCD in"=w374) -> ("error out"=w371:errorcluster, "Data Raw"=w378:T11, "Abstract_CCD out"=w372:refnum<class "Abstract_CCD.lvclass">)  [unwired: 3 in, 4 out]
            n188 = Bundle By Name(cluster=w381, "QueueAction"=DataQueue_Action."Set_Dark", "Data_Dark"=w378) -> (w382:T6)
            n189 = Enqueue Element(queue=w380, element=w382) -> (queue out=w377:refnum<queue>)  [unwired: 2 in, 2 out]
            n190 = Bundle By Name(cluster=w376, "Abstract_CCD.lvclass"=w372) -> (w375:T5)
            n191 = property on="Measure:\nRecord_Darkspec" class="Bool (strict)"(error in=w371, "Value"=FALSE ("Record_Darkspec")) -> (error out=w369:errorcluster)  [unwired: 1 in, 1 out]
            n192 = property on="SpectralStability:\nRecord_Darkspec" class="Bool (strict)"(error in=w369, "Value"=FALSE ("SpectralStability:\nRecord_Darkspec")) -> (error out=w368:errorcluster)  [unwired: 1 in, 1 out]
          }
          frame "Spectrometer_SetReference" {
            w396 = T6 {"QueueAction"=enum."TimeOut", "Data"=[], "Data_Raw"=[], "Data_Dark"=[], "Data_Ref"=[], "Device Information"=[], "Numeric Control"=0.0, "Boolean"=FALSE, "Wavelength"=[], "Time"=[], "Time Stamp"=timestamp(0 s since 1904-01-01), "Numeric Control 2"=0.0, "TabControl"=enum."Measure"}  # DataQueue
            n193 = Unbundle By Name(w391) -> ("Abstract_CCD.lvclass"=w388:refnum<class "Abstract_CCD.lvclass">)
            n194 = call-dynamic "Measure.vi"("error in (no error)"=w389, "Abstract_CCD in"=w388) -> ("error out"=w386:errorcluster, "Data Raw"=w393:T11, "Abstract_CCD out"=w387:refnum<class "Abstract_CCD.lvclass">)  [unwired: 3 in, 4 out]
            n195 = Bundle By Name(cluster=w396, "QueueAction"=DataQueue_Action."Set_Ref", "Data_Ref"=w393) -> (w397:T6)
            n196 = Enqueue Element(queue=w395, element=w397) -> (queue out=w392:refnum<queue>)  [unwired: 2 in, 2 out]
            n197 = Bundle By Name(cluster=w391, "Abstract_CCD.lvclass"=w387) -> (w390:T5)
            n198 = property on="Record RefSpec" class="Bool (strict)"(error in=w386, "Value"=FALSE ("Record RefSpec")) -> (error out=w385:errorcluster)  [unwired: 1 in, 1 out]
          }
          frame "Spectrometer_SetTriggerMode" {
            n199 = Unbundle By Name(w402) -> ("Abstract_CCD.lvclass"=w407:refnum<class "Abstract_CCD.lvclass">)
            n200 = Unbundle By Name(w406) -> ("Numeric 1"=w404:dbl)
            n201 = call-dynamic "Set_TriggerMode.vi"("error in (no error)"=w405, "Trigger Mode"=w404, "Abstract_CCD in"=w407) -> ("error out"=w403:errorcluster, "Abstract_CCD out"=w401:refnum<class "Abstract_CCD.lvclass">)  [unwired: 7 in]
            n202 = Bundle By Name(cluster=w402, "Abstract_CCD.lvclass"=w401) -> (w400:T5)
          }
          frame "Spectrometer_DeviceInformation" {
            w415 = T6 {"QueueAction"=enum."TimeOut", "Data"=[], "Data_Raw"=[], "Data_Dark"=[], "Data_Ref"=[], "Device Information"=[], "Numeric Control"=0.0, "Boolean"=FALSE, "Wavelength"=[], "Time"=[], "Time Stamp"=timestamp(0 s since 1904-01-01), "Numeric Control 2"=0.0, "TabControl"=enum."Measure"}  # DataQueue
            n203 = Unbundle By Name(w409) -> ("Abstract_CCD.lvclass"=w417:refnum<class "Abstract_CCD.lvclass">)
            n204 = call-dynamic "Get_DeviceInformation.vi"("error in (no error)"=w416, "Abstract_CCD in"=w417) -> ("error out"=w411:errorcluster, "Array"=w418:string[])  [unwired: 7 in, 1 out]
            n205 = Bundle By Name(cluster=w415, "QueueAction"=DataQueue_Action."Transfer_Settings", "Device Information"=w418) -> (w413:T6)
            n206 = Enqueue Element(queue=w414, element=w413, error in (no error)=w411) -> (queue out=w412:refnum<queue>, error out=w410:errorcluster)  [unwired: 1 in, 1 out]
          }
          frame "Arduino_Init" {
            n207 = Unbundle By Name(w429) -> ("SpinCoater.lvclass"=w428:refnum<class "SpinCoater.lvclass">)
            n208 = call-dynamic "Init.vi"("error in (no error)"=w427, "Variant"="Port Arduino", "SpinCoater in"=w428) -> ("error out"=w424:errorcluster, "SpinCoater out"=w425:refnum<class "SpinCoater.lvclass">)  [unwired: 7 in]
            n209 = call-dynamic "IsInit.vi"("error in (no error)"=w424, "SpinCoater in"=w425) -> ("error out"=w421:errorcluster, "Init"=w422:bool, "SpinCoater out"=w423:refnum<class "SpinCoater.lvclass">)  [unwired: 7 in]
            n210 = property on="Arduino" class="Bool (strict)"("Value"=w422) -> ()  [unwired: 2 in, 2 out]
            n211 = case shown="True" w422 {
              tunnel: w432 -> [w436 w445]
              tunnel: [w436 w439] -> w431
              tunnel: [w435 w438] -> w430
              tunnel: w421 -> [w435 w442]
              frame False {
              }
              frame True {
                w446 = T9 {"QueueAction"=enum."TimeOut", "Numeric 1"=0.0, "Numeric 2"=0.0, "Boolean 1"=FALSE, "Boolean 2"=FALSE, "Spin Program"=[], "Spin Prg v07"=[], "Time Stamp"=timestamp(0 s since 1904-01-01), "TabControl"=enum."Measure"}  # Device Queue
                n212 = property on="Program Spin Coater" class="Arr (strict)"() -> ("Value"=w437:T2)  [unwired: 2 in, 2 out]
                n213 = property on="Seconds to Spin" class="DigNum (strict)"() -> ("Value"=w441:dbl[unit])  [unwired: 2 in, 2 out]
                n214 = node(w441) -> (w440:dbl)
                n215 = Bundle By Name(cluster=w446, "QueueAction"=DeviceQueue_Action."Arduino_LoadProgram", "Spin Prg v07"=w437, "Numeric 1"=w440) -> (w444:T9)
                n216 = Enqueue Element(queue=w445, element=w444, error in (no error)=w442) -> (queue out=w439:refnum<queue>, error out=w438:errorcluster)  [unwired: 1 in, 1 out]
              }
            }
            n217 = Bundle By Name(cluster=w429, "SpinCoater.lvclass"=w423) -> (w433:T5)
          }
          frame "Arduino_Close" {
            n218 = Unbundle By Name(w449) -> ("SpinCoater.lvclass"=w457:refnum<class "SpinCoater.lvclass">)
            n219 = property on="Arduino" class="Bool (strict)"() -> (error out=w451:errorcluster, "Value"=w450:bool)  [unwired: 2 in, 1 out]
            n220 = property on="Arduino" class="Bool (strict)"(error in=w451, "Value"=FALSE ("Arduino")) -> ()  [unwired: 1 in, 2 out]
            n221 = case shown="False" w450 {
              tunnel: w457 -> [w458 w463]
              tunnel: w456 -> [w459 w462]
              tunnel: [w459 w461] -> w455
              tunnel: [w458 w460] -> w448
              frame False {
              }
              frame True {
                n222 = call-dynamic "Close.vi"("error in (no error)"=w462, "SpinCoater in"=w463) -> ("error out"=w461:errorcluster, "SpinCoater out"=w460:refnum<class "SpinCoater.lvclass">)  [unwired: 8 in]
              }
            }
            n223 = Bundle By Name(cluster=w449, "SpinCoater.lvclass"=w448) -> (w447:T5)
          }
          frame "Arduino_LoadProgram" {
            n224 = Unbundle By Name(w473) -> ("Spin Prg v07"=w464:T2, "Numeric 1"=w472:dbl)
            n225 = Unbundle By Name(w468) -> ("SpinCoater.lvclass"=w471:refnum<class "SpinCoater.lvclass">)
            n226 = node(w472) -> (w470:dbl[unit])
            n227 = call-dynamic "Program_Load_v02.vi"("error in (no error)"=w469, "Time Start"=w470, "Program Spin Coater"=w464, "SpinCoater in"=w471) -> ("error out"=w466:errorcluster, "SpinCoater out"=w467:refnum<class "SpinCoater.lvclass">)  [unwired: 6 in]
            n228 = Bundle By Name(cluster=w468, "SpinCoater.lvclass"=w467) -> (w465:T5)
          }
          frame "Arduino_StartProgram" {
            n229 = Unbundle By Name(w481) -> ("SpinCoater.lvclass"=w478:refnum<class "SpinCoater.lvclass">)
            n230 = call-dynamic "Program_Run.vi"("error in (no error)"=w477, "SpinCoater in"=w478) -> ("error out"=w476:errorcluster)  [unwired: 8 in, 1 out]
            n231 = property on="Action" class="Str"("Value"="Measuring" ("Action")) -> ()  [unwired: 2 in, 2 out]
          }
          frame "Arduino_SetSpeed" {
            n232 = Unbundle By Name(w490) -> ("SpinCoater.lvclass"=w486:refnum<class "SpinCoater.lvclass">)
            n233 = Unbundle By Name(w489) -> ("Numeric 1"=w488:dbl)
            n234 = To Unsigned Long Integer(number=w488) -> (unsigned 32bit integer=w484:u32)
            n235 = call-dynamic "Debug_SetSpeed.vi"("error in (no error)"=w485, "Speed"=w484, "SpinCoater in"=w486) -> ("error out"=w483:errorcluster)  [unwired: 7 in, 1 out]
          }
          frame "Arduino_SetMillis" {
            n236 = Unbundle By Name(w496) -> ("SpinCoater.lvclass"=w495:refnum<class "SpinCoater.lvclass">)
            n237 = Unbundle By Name(w498) -> ("Numeric 1"=w500:dbl)
            n238 = To Unsigned Long Integer(number=w500) -> (unsigned 32bit integer=w492:u32)
            n239 = call-dynamic "Debug_SetMillis.vi"("error in (no error)"=w494, "Milliseconds"=w492, "SpinCoater in"=w495) -> ("error out"=w493:errorcluster)  [unwired: 7 in, 1 out]
          }
          frame "Arduino_StopSpin" {
            n240 = Unbundle By Name(w504) -> ("SpinCoater.lvclass"=w503:refnum<class "SpinCoater.lvclass">)
            n241 = call-dynamic "Stop_Spin.vi"("error in (no error)"=w502, "SpinCoater in"=w503) -> ("error out"=w501:errorcluster)  [unwired: 8 in, 1 out]
          }
          frame "Measure_Stop" {
            w513 = T6 {"QueueAction"=enum."TimeOut", "Data"=[], "Data_Raw"=[], "Data_Dark"=[], "Data_Ref"=[], "Device Information"=[], "Numeric Control"=0.0, "Boolean"=FALSE, "Wavelength"=[], "Time"=[], "Time Stamp"=timestamp(0 s since 1904-01-01), "Numeric Control 2"=0.0, "TabControl"=enum."Measure"}  # DataQueue
            n242 = Bundle By Name(cluster=w513, "QueueAction"=DataQueue_Action."Stop_Measurement") -> (w514:T6)
            n243 = Enqueue Element(queue=w511, element=w514, error in (no error)=w508) -> (queue out=w510:refnum<queue>, error out=w507:errorcluster)  [unwired: 1 in, 1 out]
          }
          frame "Measure_InSitu" {
            w555 = T9 {"QueueAction"=enum."TimeOut", "Numeric 1"=0.0, "Numeric 2"=0.0, "Boolean 1"=FALSE, "Boolean 2"=FALSE, "Spin Program"=[], "Spin Prg v07"=[], "Time Stamp"=timestamp(0 s since 1904-01-01), "TabControl"=enum."Measure"}  # Device Queue
            w562 = T9 {"QueueAction"=enum."TimeOut", "Numeric 1"=0.0, "Numeric 2"=0.0, "Boolean 1"=FALSE, "Boolean 2"=FALSE, "Spin Program"=[], "Spin Prg v07"=[], "Time Stamp"=timestamp(0 s since 1904-01-01), "TabControl"=enum."Measure"}  # Device Queue
            n244 = Bundle By Name(cluster=w562, "QueueAction"=DeviceQueue_Action."Spectrometer_SetTriggerMode", "Numeric 1"=1.0) -> (w560:T9)
            n245 = Bundle By Name(cluster=w555, "QueueAction"=DeviceQueue_Action."Spectrometer_DeviceInformation") -> (w552:T9)
            n246 = Bundle By Name(cluster=w552, "QueueAction"=DeviceQueue_Action."Spectrometer_StartMeasurement") -> (w548:T9)
            n247 = Enqueue Element(queue=w561, element=w560, error in (no error)=w517) -> (queue out=w557:refnum<queue>, error out=w558:errorcluster)  [unwired: 1 in, 1 out]
            n248 = property on="Frames" class="DigNum (strict)"() -> ("Value"=w518:i32)  [unwired: 2 in, 2 out]
            n249 = Bundle By Name(cluster=w548, "QueueAction"=DeviceQueue_Action."Arduino_StartProgram") -> (w543:T9)
            n250 = Enqueue Element(queue=w557, element=w552, error in (no error)=w558) -> (queue out=w554:refnum<queue>, error out=w553:errorcluster)  [unwired: 1 in, 1 out]
            n251 = Bundle By Name(cluster=w543, "QueueAction"=DeviceQueue_Action."Spectrometer_GetData", "Numeric 1"="Dividider Get Spectra") -> (w538:T9)
            n252 = Divide(x=w518, y="Dividider Get Spectra") -> (x/y=w550:dbl)
            n253 = Round Toward +Infinity(x=w550) -> (ceil(x): smallest int >= x=w549:dbl)
            n254 = Enqueue Element(queue=w554, element=w548, error in (no error)=w553) -> (queue out=w547:refnum<queue>, error out=w546:errorcluster)  [unwired: 1 in, 1 out]
            n255 = Enqueue Element(queue=w547, element=w543, error in (no error)=w546) -> (queue out=w544:refnum<queue>, error out=w541:errorcluster)  [unwired: 1 in, 1 out]
            n256 = for {
              N: w549 -> [_]
              shift-right: [w565] -> w540
              shift-left: w544 -> [w569]
              tunnel: w538 -> [w566]
              shift-right: [w567] -> w539
              shift-left: w541 -> [w568]
              n257 = Enqueue Element(queue=w569, element=w566, error in (no error)=w568) -> (queue out=w565:refnum<queue>, error out=w567:errorcluster)  [unwired: 1 in, 1 out]
            }
            n258 = Bundle By Name(cluster=w538, "QueueAction"=DeviceQueue_Action."Spectrometer_StopMeasurement") -> (w534:T9)
            n259 = property on="Measure_FramesSpectrometer" class="DigNum (strict)"() -> ("Value"=w520:dbl)  [unwired: 2 in, 2 out]
            n260 = Bundle By Name(cluster=w534, "QueueAction"=DeviceQueue_Action."Measure_Stop") -> (w527:T9)
            n261 = Enqueue Element(queue=w540, element=w534, error in (no error)=w539) -> (queue out=w535:refnum<queue>, error out=w536:errorcluster)  [unwired: 1 in, 1 out]
            n262 = Bundle By Name(cluster=w527, "QueueAction"=DeviceQueue_Action."Spectrometer_SetTriggerMode", "Numeric 1"=0.0) -> (w522:T9)
            n263 = Enqueue Element(queue=w535, element=w527, error in (no error)=w536) -> (queue out=w530:refnum<queue>, error out=w531:errorcluster)  [unwired: 1 in, 1 out]
            n264 = Bundle By Name(cluster=w522, "QueueAction"=DeviceQueue_Action."Spectrometer_SetFrames", "Numeric 1"=w520) -> (w519:T9)
            n265 = Enqueue Element(queue=w530, element=w522, error in (no error)=w531) -> (queue out=w529:refnum<queue>, error out=w528:errorcluster)  [unwired: 1 in, 1 out]
            n266 = Enqueue Element(queue=w529, element=w519, error in (no error)=w528) -> (queue out=w523:refnum<queue>, error out=w524:errorcluster)  [unwired: 1 in, 1 out]
          }
          frame "Measure_InSituAdvanced" {
            w652 = T9 {"QueueAction"=enum."TimeOut", "Numeric 1"=0.0, "Numeric 2"=0.0, "Boolean 1"=FALSE, "Boolean 2"=FALSE, "Spin Program"=[], "Spin Prg v07"=[], "Time Stamp"=timestamp(0 s since 1904-01-01), "TabControl"=enum."Measure"}  # Device Queue
            n267 = property on="Dividider Get Spectra" class="DigNum (strict)"() -> ("Value"=w611:u32)  [unwired: 2 in, 2 out]
            n268 = Bundle By Name(cluster=w652, "QueueAction"=DeviceQueue_Action."Spectrometer_SetTriggerMode", "Numeric 1"=1.0) -> (w607:T9)
            n269 = Bundle By Name(cluster=w607, "QueueAction"=DeviceQueue_Action."Spectrometer_DeviceInformation") -> (w644:T9)
            n270 = Bundle By Name(cluster=w644, "QueueAction"=DeviceQueue_Action."Spectrometer_StartMeasurement") -> (w640:T9)
            n271 = Enqueue Element(queue=w651, element=w607, error in (no error)=w612) -> (queue out=w648:refnum<queue>, error out=w649:errorcluster)  [unwired: 1 in, 1 out]
            n272 = Bundle By Name(cluster=w640, "QueueAction"=DeviceQueue_Action."Arduino_StartProgram") -> (w635:T9)
            n273 = property on="Frames" class="DigNum (strict)"() -> ("Value"=w613:i32)  [unwired: 2 in, 2 out]
            n274 = Unbundle By Name(w594) -> ("Time Stamp"=w593:timestamp)
            n275 = Enqueue Element(queue=w648, element=w644, error in (no error)=w649) -> (queue out=w646:refnum<queue>, error out=w645:errorcluster)  [unwired: 1 in, 1 out]
            n276 = Divide(x=w613, y=w611) -> (x/y=w642:dbl)
            n277 = Bundle By Name(cluster=w635, "QueueAction"=DeviceQueue_Action."Spectrometer_GetData", "Numeric 1"=w611) -> (w630:T9)
            n278 = Round Toward +Infinity(x=w642) -> (ceil(x): smallest int >= x=w641:dbl)
            n279 = Enqueue Element(queue=w646, element=w640, error in (no error)=w645) -> (queue out=w639:refnum<queue>, error out=w638:errorcluster)  [unwired: 1 in, 1 out]
            n280 = Enqueue Element(queue=w639, element=w635, error in (no error)=w638) -> (queue out=w636:refnum<queue>, error out=w633:errorcluster)  [unwired: 1 in, 1 out]
            n281 = Bundle By Name(cluster=w630, "QueueAction"=DeviceQueue_Action."Spectrometer_StopMeasurement") -> (w626:T9)
            n282 = for {
              N: w641 -> [_]
              shift-right: [w702] -> w632
              shift-left: w636 -> [w706]
              tunnel: w630 -> [w703]
              shift-right: [w704] -> w631
              shift-left: w633 -> [w705]
              n283 = Enqueue Element(queue=w706, element=w703, error in (no error)=w705) -> (queue out=w702:refnum<queue>, error out=w704:errorcluster)  [unwired: 1 in, 1 out]
            }
            n284 = property on="Measure_FramesSpectrometer" class="DigNum (strict)"() -> ("Value"=w614:dbl)  [unwired: 2 in, 2 out]
            n285 = property on="periodic time" class="DigNum (strict)"() -> ("Value"=w606:dbl[unit])  [unwired: 2 in, 2 out]
            n286 = Bundle By Name(cluster=w626, "QueueAction"=DeviceQueue_Action."Measure_Stop") -> (w619:T9)
            n287 = property on="Duration after" class="DigNum (strict)"() -> ("Value"=w605:dbl[unit])  [unwired: 2 in, 2 out]
            n288 = node(w606) -> (w573:dbl)
            n289 = property on="periodic time" class="DigNum (strict)"() -> ("Value"=w604:dbl[unit])  [unwired: 2 in, 2 out]
            n290 = Bundle By Name(cluster=w619, "QueueAction"=DeviceQueue_Action."Spectrometer_SetTriggerMode", "Numeric 1"=0.0) -> (w616:T9)
            n291 = Enqueue Element(queue=w632, element=w626, error in (no error)=w631) -> (queue out=w627:refnum<queue>, error out=w628:errorcluster)  [unwired: 1 in, 1 out]
            n292 = node(w605) -> (w599:dbl)
            n293 = Bundle By Name(cluster=w616, "QueueAction"=DeviceQueue_Action."Spectrometer_SetFrames", "Numeric 1"=w614) -> (w596:T9)
            n294 = Enqueue Element(queue=w627, element=w619, error in (no error)=w628) -> (queue out=w622:refnum<queue>, error out=w623:errorcluster)  [unwired: 1 in, 1 out]
            n295 = node(w604) -> (w598:dbl)
            n296 = Bundle By Name(cluster=w596, "QueueAction"=DeviceQueue_Action."Wait", "Numeric 1"=w573) -> (w575:T9)
            n297 = Enqueue Element(queue=w622, element=w616, error in (no error)=w623) -> (queue out=w621:refnum<queue>, error out=w620:errorcluster)  [unwired: 1 in, 1 out]
            n298 = Not Equal To 0?(x=w598) -> (x != 0?=w602:bool)
            n299 = Not Equal To 0?(x=w599) -> (x != 0?=w603:bool)
            n300 = Divide(x=w599, y=w598) -> (x/y=w600:dbl)
            n301 = Bundle By Name(cluster=w575, "QueueAction"=DeviceQueue_Action."Spectrometer_MeasureAdvanced", "Time Stamp"=w593) -> (w574:T9)
            n302 = And(x=w603, y=w602) -> (x .and. y?=w601:bool)
            n303 = Round Toward +Infinity(x=w600) -> (ceil(x): smallest int >= x=w597:dbl)
            n304 = Enqueue Element(queue=w621, element=w596, error in (no error)=w620) -> (queue out=w610:refnum<queue>, error out=w609:errorcluster)  [unwired: 1 in, 1 out]
            n305 = Bundle By Name(cluster=w574, "QueueAction"=DeviceQueue_Action."Arduino_SetSpeed", "Numeric 1"=1500.0) -> (w588:T9)
            n306 = Bundle By Name(cluster=w588, "Numeric 1"=0.0) -> (w579:T9)
            n307 = property on="Measure_FrameRate" class="DigNum (strict)"() -> ("Value"=w585:dbl[unit])  [unwired: 2 in, 2 out]
            n308 = property on="Measure_FramesSpectrometer" class="DigNum (strict)"() -> ("Value"=w584:dbl)  [unwired: 2 in, 2 out]
            n309 = Divide(x=w584, y=w585) -> (x/y=w586:dbl[unit])
            n310 = Bundle By Name(cluster=w575, "Numeric 1"=1.0) -> (w581:T9)
            n311 = node(w586) -> (w572:dbl)
            n312 = Subtract(x=w573, y=w572) -> (x-y=w571:dbl)
            n313 = Bundle By Name(cluster=w575, "Numeric 1"=w571) -> (w570:T9)
            n314 = Round Toward +Infinity(x=w572) -> (ceil(x): smallest int >= x=w587:dbl)
            n315 = Add(x=w587, y=2.0) -> (x+y=w582:dbl)
            n316 = Bundle By Name(cluster=w581, "Numeric 1"=w582) -> (w580:T9)
            n317 = case shown="True" w601 {
              tunnel: w610 -> [w656 w658]
              tunnel: w609 -> [w655 w661]
              tunnel: w597 -> [_ w674]
              tunnel: w574 -> [_ w673]
              tunnel: w570 -> [_ w669]
              tunnel: w588 -> [_ w668]
              tunnel: w581 -> [_ w667]
              tunnel: w574 -> [_ w666]
              tunnel: w580 -> [_ w665]
              tunnel: w579 -> [_ w664]
              tunnel: [w655 w663] -> w578
              tunnel: [w656 w662] -> w577
              tunnel: w575 -> [_ w657]
              frame False {
              }
              frame True {
                n318 = Enqueue Element(queue=w658, element=w657, error in (no error)=w661) -> (queue out=w659:refnum<queue>, error out=w660:errorcluster)  [unwired: 1 in, 1 out]
                n319 = for {
                  N: w674 -> [_]
                  shift-right: [w695] -> w671
                  shift-left: w659 -> [w701]
                  shift-right: [w694] -> w670
                  shift-left: w660 -> [w700]
                  tunnel: w673 -> [w699]
                  tunnel: w669 -> [w696]
                  n320 = Enqueue Element(queue=w701, element=w699, error in (no error)=w700) -> (queue out=w697:refnum<queue>, error out=w698:errorcluster)  [unwired: 1 in, 1 out]
                  n321 = Enqueue Element(queue=w697, element=w696, error in (no error)=w698) -> (queue out=w695:refnum<queue>, error out=w694:errorcluster)  [unwired: 1 in, 1 out]
                }
                n322 = case shown="True" "Spin at end" {
                  tunnel: w671 -> [w676 w693]
                  tunnel: w670 -> [w675 w692]
                  tunnel: w668 -> [_ w687]
                  tunnel: w667 -> [_ w686]
                  tunnel: w666 -> [_ w685]
                  tunnel: w665 -> [_ w680]
                  tunnel: w664 -> [_ w679]
                  tunnel: [w675 w678] -> w663
                  tunnel: [w676 w677] -> w662
                  frame False {
                  }
                  frame True {
                    n323 = Enqueue Element(queue=w693, element=w687, error in (no error)=w692) -> (queue out=w691:refnum<queue>, error out=w690:errorcluster)  [unwired: 1 in, 1 out]
                    n324 = Enqueue Element(queue=w691, element=w686, error in (no error)=w690) -> (queue out=w689:refnum<queue>, error out=w688:errorcluster)  [unwired: 1 in, 1 out]
                    n325 = Enqueue Element(queue=w689, element=w685, error in (no error)=w688) -> (queue out=w684:refnum<queue>, error out=w683:errorcluster)  [unwired: 1 in, 1 out]
                    n326 = Enqueue Element(queue=w684, element=w680, error in (no error)=w683) -> (queue out=w681:refnum<queue>, error out=w682:errorcluster)  [unwired: 1 in, 1 out]
                    n327 = Enqueue Element(queue=w681, element=w679, error in (no error)=w682) -> (queue out=w677:refnum<queue>, error out=w678:errorcluster)  [unwired: 1 in, 1 out]
                  }
                }
              }
            }
            "Nr After Spin" <- u16 0 ("Nr After Spin")
          }
          frame "Measure_Spectrum" {
            n328 = Unbundle By Name(w707) -> ("Time Stamp"=w708:timestamp)
            n329 = Bundle By Name(cluster=w707, "QueueAction"=DeviceQueue_Action."Spectrometer_Measure", "Time Stamp"=w708) -> (w713:T9)
            n330 = Bundle By Name(cluster=w713, "QueueAction"=DeviceQueue_Action."Measure_Stop") -> (w711:T9)
            n331 = Enqueue Element(queue=w719, element=w713, error in (no error)=w718) -> (queue out=w714:refnum<queue>, error out=w715:errorcluster)  [unwired: 1 in, 1 out]
            n332 = Enqueue Element(queue=w714, element=w711, error in (no error)=w715) -> (queue out=w710:refnum<queue>, error out=w709:errorcluster)  [unwired: 1 in, 1 out]
          }
          frame "Measure_SpectralStability" {
            n333 = Bundle By Name(cluster=w723, "QueueAction"=DeviceQueue_Action."Spectrometer_DeviceInformation") -> (w726:T9)
            n334 = property on="SpectralStability_\nFrameRate" class="DigNum (strict)"() -> ("Value"=w746:dbl[unit])  [unwired: 2 in, 2 out]
            n335 = property on="SpectralStability_\nFramesSpectrometer" class="DigNum (strict)"() -> ("Value"=w747:dbl)  [unwired: 2 in, 2 out]
            n336 = Bundle By Name(cluster=w726, "QueueAction"=DeviceQueue_Action."Spectrometer_Measure") -> (w725:T9)
            n337 = Enqueue Element(queue=w729, element=w726, error in (no error)=w728) -> (queue out=w731:refnum<queue>, error out=w730:errorcluster)  [unwired: 1 in, 1 out]
            n338 = Divide(x=w747, y=w746) -> (x/y=w741:dbl[unit])
            n339 = Unbundle By Name(w723) -> ("Numeric 1"=w722:dbl)
            n340 = Subtract(x="SpectralStability_\nPeriodicTime", y=w741) -> (x-y=w740:dbl[unit])
            n341 = Enqueue Element(queue=w731, element=w725, error in (no error)=w730) -> (queue out=w745:refnum<queue>, error out=w744:errorcluster)  [unwired: 1 in, 1 out]
            n342 = node(w740) -> (w739:dbl)
            n343 = Decrement(x=w722) -> (x-1=w721:dbl)
            n344 = Bundle By Name(cluster=w725, "QueueAction"=DeviceQueue_Action."Wait", "Numeric 1"=w739) -> (w735:T9)
            n345 = for {
              N: w721 -> [_]
              shift-right: [w751] -> w738
              shift-left: w745 -> [w757]
              shift-right: [w750] -> w737
              shift-left: w744 -> [w756]
              tunnel: w735 -> [w753]
              tunnel: w725 -> [w752]
              n346 = Enqueue Element(queue=w757, element=w753, error in (no error)=w756) -> (queue out=w755:refnum<queue>, error out=w754:errorcluster)  [unwired: 1 in, 1 out]
              n347 = Enqueue Element(queue=w755, element=w752, error in (no error)=w754) -> (queue out=w751:refnum<queue>, error out=w750:errorcluster)  [unwired: 1 in, 1 out]
            }
            n348 = Bundle By Name(cluster=w735, "QueueAction"=DeviceQueue_Action."Measure_Stop") -> (w734:T9)
            n349 = Enqueue Element(queue=w738, element=w734, error in (no error)=w737) -> (queue out=w732:refnum<queue>, error out=w733:errorcluster)  [unwired: 1 in, 1 out]
          }
        }
      }
      frame Error {
        w762 = T12 4 items=["no dialog", "OK message", "continue or stop message", "OK message + warnings", "continue/stop + warnings"] ("type of dialog (OK msg:1)")
        n350 = call <vilib>:"General Error Handler.vi"("type of dialog (OK msg:1)"=w762, "error in (no error)"=w763) -> ("error out"=w761:errorcluster)  [unwired: 9 in, 4 out]
        n351 = call <vilib>:"Clear Errors.vi"("error in (no error)"=w761) -> ("error out"=w760:errorcluster)  [unwired: 5 in, 1 out]
      }
    }
  }
  n352 = while {
    shift-right: [w765] -> _
    shift-left: w8 -> [w771]
    shift-right: [w766] -> _
    shift-left: w7 -> [w770]
    shift-right: [w767] -> _
    shift-left: w6 -> [w769]
    stop <- w768 stop-if-true
    # "Consumer Data"
    n353 = case shown="No Error" w771 {
      selector: w771 -> [w782 w1469]
      tunnel: w770 -> [w781 w1470]
      tunnel: w769 -> [w779 w1467]
      tunnel: [w778 _] -> w768
      tunnel: [w777 w1467] -> w767
      tunnel: [w776 w1470] -> w766
      tunnel: [w774 w1468] -> w765
      frame No Error {
        n354 = Dequeue Element(queue=w781, error in (no error)=w782) -> (queue out=w775:refnum<queue>, element=w772:T6, error out=w773:errorcluster)  [unwired: 1 in, 1 out]
        n355 = Unbundle By Name(w772) -> ("QueueAction"=w780:T7)
        n356 = case shown="\"Measure_InSituSpinCoating\"" w780 {
          tunnel: w779 -> [w783 w788 w794 w967 w1072 w1174 w1382 w1418 w1427 w1449 w1462]
          tunnel: [_ TRUE _ _ _ _ _ _ _ _ _] -> w778
          tunnel: [w783 w788 w794 w967 w1072 w1165 w1382 w1422 w1441 w1448 w1462] -> w777
          tunnel: [w785 w787 w804 w973 w1078 w1158 w1405 w1423 w1442 w1445 w1464] -> w776
          tunnel: w775 -> [w785 w787 w802 w974 w1079 w1169 w1405 w1423 w1442 w1445 w1464]
          tunnel: [w784 w786 w803 w972 w1077 w1159 w1404 w1424 w1443 w1446 w1463] -> w774
          tunnel: w773 -> [w784 w786 w801 w975 w1080 w1168 w1404 w1424 w1443 w1446 w1463]
          tunnel: w772 -> [_ _ w796 _ _ w1161 w1395 w1425 w1444 w1447 w1453]
          frame "TimeOut", Default {
          }
          frame "Close_Program" {
          }
          frame "Measure_InSituSpinCoating" {
            w799 = T6 {"QueueAction"=enum."TimeOut", "Data"=[], "Data_Raw"=[], "Data_Dark"=[], "Data_Ref"=[], "Device Information"=[], "Numeric Control"=0.0, "Boolean"=FALSE, "Wavelength"=[], "Time"=[], "Time Stamp"=timestamp(0 s since 1904-01-01), "Numeric Control 2"=0.0, "TabControl"=enum."Measure"}  # DataQueue
            n357 = property on="Seconds to\nSpin Start" class="DigNum (strict)"() -> ("Value"=w791:dbl[unit])  [unwired: 2 in, 2 out]
            n358 = Unbundle By Name(w796) -> ("Time Stamp"=w795:timestamp)
            n359 = node(w791) -> (w790:dbl)
            n360 = Obtain Queue(name (unnamed)="Temp", element data type=w799) -> (queue out=w798:refnum<queue>)  [unwired: 3 in, 2 out]
            n361 = while {
              shift-right: [w812] -> w804
              shift-left: w802 -> [w821]
              shift-right: [w813] -> w803
              shift-left: w801 -> [w820]
              shift-right: [w814] -> w797
              shift-left: w798 -> [w815]
              tunnel: w795 -> [w808]
              shift-right: [w809] -> _
              shift-left: string[] [] ("Device Information") -> [w810]
              border: FALSE -> [_]
              tunnel: w790 -> [w805]
              stop <- w811 stop-if-true
              n362 = Dequeue Element(queue=w821, error in (no error)=w820) -> (queue out=w816:refnum<queue>, element=w818:T6, error out=w817:errorcluster)  [unwired: 1 in, 1 out]
              n363 = Unbundle By Name(w818) -> ("QueueAction"=w819:T7)
              n364 = feedback #1() -> (w807:bool)
              n365 = case shown="Default" w819 {
                tunnel: w818 -> [w829 w838 _ w884 w921 w965]
                tunnel: w817 -> [w828 w839 w845 w881 w912 w962]
                tunnel: w816 -> [w824 w840 w844 w880 w920 w963]
                tunnel: w815 -> [w827 w835 w846 w875 w909 w966]
                tunnel: [w826 w835 w841 w872 w909 w966] -> w814
                tunnel: [w825 w836 w843 w871 w910 w962] -> w813
                tunnel: [w824 w837 w842 w870 w920 w963] -> w812
                tunnel: [_ TRUE TRUE TRUE _ _] -> w811
                tunnel: w810 -> [w823 w833 w853 w882 w907 _]
                tunnel: [w823 w833 w853 w882 w907 w964] -> w809
                tunnel: w808 -> [_ _ _ w883 w922 _]
                tunnel: w807 -> [w822 w832 w852 w869 w905 w961]
                tunnel: [w822 w832 w852 w869 TRUE w961] -> w806
                tunnel: w805 -> [_ _ _ w866 _ _]
                frame Default {
                  n366 = Enqueue Element(queue=w827, element=w829, error in (no error)=w828) -> (queue out=w826:refnum<queue>, error out=w825:errorcluster)  [unwired: 1 in, 1 out]
                }
                frame "Close_Program" {
                  n367 = Enqueue Element At Opposite End(queue=w840, element=w838, error in (no error)=w839) -> (queue out=w837:refnum<queue>, error out=w836:errorcluster)  [unwired: 1 in, 1 out]
                  n368 = property on="Time.spin" class="Ref (strict)"() -> ("Value"=w830:refnum<file>)  [unwired: 2 in, 2 out]
                  n369 = property on="Meas.spin" class="Ref (strict)"() -> ("Value"=w831:refnum<file>)  [unwired: 2 in, 2 out]
                  n370 = Close File(refnum=w831) -> ()  [unwired: 1 in, 2 out]
                  n371 = Close File(refnum=w830) -> ()  [unwired: 1 in, 2 out]
                }
                frame "Abort" {
                  n372 = property on="Time.spin" class="Ref (strict)"() -> ("Value"=w850:refnum<file>)  [unwired: 2 in, 2 out]
                  n373 = Get Queue Status(queue=w846) -> (queue out=w847:refnum<queue>, # elements in queue=w848:i32)  [unwired: 2 in, 6 out]
                  n374 = property on="Meas.spin" class="Ref (strict)"() -> ("Value"=w851:refnum<file>)  [unwired: 2 in, 2 out]
                  n375 = Close File(refnum=w851) -> ()  [unwired: 1 in, 2 out]
                  n376 = Close File(refnum=w850) -> ()  [unwired: 1 in, 2 out]
                  n377 = for {
                    N: w848 -> [_]
                    shift-right: [w860] -> w841
                    shift-left: w847 -> [w861]
                    shift-right: [w857] -> w842
                    shift-left: w844 -> [w858]
                    shift-right: [w855] -> w843
                    shift-left: w845 -> [w856]
                    n378 = Dequeue Element(queue=w861) -> (queue out=w860:refnum<queue>, element=w859:T6)  [unwired: 2 in, 2 out]
                    n379 = Enqueue Element(queue=w858, element=w859, error in (no error)=w856) -> (queue out=w857:refnum<queue>, error out=w855:errorcluster)  [unwired: 1 in, 1 out]
                  }
                  n380 = property on="StartMeasurement_Button" class="Bool (strict)"("Value"=FALSE ("StartMeasurement_Button")) -> ()  [unwired: 2 in, 2 out]
                }
                frame "Stop_Measurement" {
                  n381 = property on="Automatically \nadjust count" class="Bool (strict)"() -> ("Value"=w863:bool)  [unwired: 2 in, 2 out]
                  n382 = property on="Reset Count\nafter Spin Coating" class="Bool (strict)"() -> ("Value"=w864:bool)  [unwired: 2 in, 2 out]
                  n383 = Or(x=w863, y=w864) -> (x .or. y?=w862:bool)
                  n384 = Bundle By Name(cluster=w884, "QueueAction"=DataQueue_Action."Save_InSitu", "Time Stamp"=w883, "Device Information"=w882, "Numeric Control"=w866) -> (w879:T6)
                  n385 = case shown="True" w862 {
                    frame False {
                    }
                    frame True {
                      n386 = property on="Spectra \nCount" class="DigNum (strict)"("Value"=u16 0 ("Spectra Count")) -> ()  [unwired: 2 in, 2 out]
                    }
                  }
                  n387 = Enqueue Element(queue=w880, element=w879, error in (no error)=w881) -> (queue out=w877:refnum<queue>, error out=w876:errorcluster)  [unwired: 1 in, 1 out]
                  n388 = Get Queue Status(queue=w875) -> (queue out=w873:refnum<queue>, # elements in queue=w874:i32)  [unwired: 2 in, 6 out]
                  n389 = property on="Time.spin" class="Ref (strict)"() -> ("Value"=w867:refnum<file>)  [unwired: 2 in, 2 out]
                  n390 = property on="StartMeasurement_Button" class="Bool (strict)"("Value"=FALSE ("StartMeasurement_Button")) -> ()  [unwired: 2 in, 2 out]
                  n391 = property on="Meas.spin" class="Ref (strict)"() -> ("Value"=w868:refnum<file>)  [unwired: 2 in, 2 out]
                  n392 = for {
                    N: w874 -> [_]
                    shift-right: [w892] -> w872
                    shift-left: w873 -> [w893]
                    shift-right: [w889] -> w870
                    shift-left: w877 -> [w890]
                    shift-right: [w887] -> w871
                    shift-left: w876 -> [w888]
                    n393 = Dequeue Element(queue=w893) -> (queue out=w892:refnum<queue>, element=w891:T6)  [unwired: 2 in, 2 out]
                    n394 = Enqueue Element(queue=w890, element=w891, error in (no error)=w888) -> (queue out=w889:refnum<queue>, error out=w887:errorcluster)  [unwired: 1 in, 1 out]
                  }
                  n395 = Close File(refnum=w868) -> ()  [unwired: 1 in, 2 out]
                  n396 = Close File(refnum=w867) -> ()  [unwired: 1 in, 2 out]
                }
                frame "Spectrometer_Measure" {
                  w895 = FALSE ("prepend array or string size? (T)")
                  w908 = enum16{"start", "end", "current"}."end" ("from (0:start)")
                  n397 = Unbundle By Name(w921) -> ("Data_Raw"=w917:T11, "Time"=w911:dbl[])
                  n398 = Index Array(array=w917, index=0) -> (element=w916:T14)
                  n399 = To Unsigned Long Integer(number=w911) -> (unsigned 32bit integer=w897:u32[])
                  n400 = Unbundle By Name(w916) -> ("Image"=w894:dbl[][][])
                  n401 = case shown="False" w905 {
                    tunnel: w922 -> [w954 _]
                    tunnel: w912 -> [w949 w960]
                    tunnel: [w935 w960] -> w899
                    tunnel: [w923 _] -> w900
                    tunnel: [w934 w959] -> w902
                    tunnel: [w924 w958] -> w901
                    tunnel: w894 -> [w932 _]
                    frame False {
                      w944 = T13."open or create" ("operation (0:open)")
                      w943 = "_" ("string")
                      n402 = property on="Measure_FileName" class="Str"() -> ("Value"=w952:string)  [unwired: 2 in, 2 out]
                      n403 = Concatenate Strings(w952, "_meas.spin" ("string")) -> (w955:string)
                      n404 = Concatenate Strings(w952, "_time.spin" ("string")) -> (w947:string)
                      n405 = Format Date/Time String(time format string (%c)="%Y%m%d_%H%M%S", seconds (now)=w954) -> (date/time string=w948:string)  [unwired: 1 in]
                      n406 = property on="Measure_SavePath" class="Path"() -> ("Value"=w926:path)  [unwired: 2 in, 2 out]
                      n407 = Concatenate Strings(w948, w943, w955) -> (w953:string)
                      n408 = Concatenate Strings(w948, w943, w947) -> (w946:string)
                      n409 = property on="Frames" class="DigNum (strict)"() -> ("Value"=w925:i32)  [unwired: 2 in, 2 out]
                      n410 = Build Path(base path=w926, name or relative path=w953) -> (appended path=w950:path)
                      n411 = Build Path(base path=w926, name or relative path=w946) -> (appended path=w945:path)
                      n412 = Array Size(array=w932) -> (size(s)=w931:i32[])
                      n413 = Open/Create/Replace File(file path (use dialog)=w950, error in=w949, operation (0:open)=w944) -> (refnum out=w942:refnum<file>, error out=w941:errorcluster)  [unwired: 3 in, 1 out]
                      "Meas.spin" <- w942
                      n414 = Open/Create/Replace File(file path (use dialog)=w945, error in=w949, operation (0:open)=w944) -> (refnum out=w940:refnum<file>, error out=w939:errorcluster)  [unwired: 3 in, 1 out]
                      n415 = Write to Binary File(file (use dialog)=w942, data=w925, error in=w941) -> (refnum out=w938:refnum<file>, error out=w937:errorcluster)  [unwired: 3 in, 1 out]
                      n416 = Index Array(array=w931, index #1=2 ("index"), index #2=1 ("index")) -> (element #1=w927:i32, element #2=w928:i32)
                      n417 = Write to Binary File(file (use dialog)=w940, data=w925, error in=w939) -> (refnum out=w924:refnum<file>, error out=w923:errorcluster)  [unwired: 3 in, 1 out]
                      "Time.spin" <- w924
                      n418 = Write to Binary File(file (use dialog)=w938, data=w928, error in=w937) -> (refnum out=w933:refnum<file>, error out=w936:errorcluster)  [unwired: 3 in, 1 out]
                      n419 = Write to Binary File(file (use dialog)=w933, data=w927, error in=w936) -> (refnum out=w934:refnum<file>, error out=w935:errorcluster)  [unwired: 3 in, 1 out]
                    }
                    frame True {
                      n420 = property on="Time.spin" class="Ref (strict)"() -> ("Value"=w958:refnum<file>)  [unwired: 2 in, 2 out]
                      n421 = property on="Meas.spin" class="Ref (strict)"() -> ("Value"=w959:refnum<file>)  [unwired: 2 in, 2 out]
                    }
                  }
                  n422 = To Unsigned Word Integer(number=w894) -> (unsigned 16bit integer=w896:u16[][][])
                  n423 = Merge Errors(w899, w900) -> (w898:errorcluster)
                  n424 = Set File Position(refnum=w902, from (0:start)=w908, error in=w898) -> (refnum out=w914:refnum<file>, error out=w913:errorcluster)  [unwired: 1 in]
                  n425 = Set File Position(refnum=w901, from (0:start)=w908, error in=w898) -> (refnum out=w919:refnum<file>, error out=w918:errorcluster)  [unwired: 1 in]
                  n426 = Write to Binary File(file (use dialog)=w919, data=w897, error in=w918, 5:w895) -> (error out=w903:errorcluster)  [unwired: 2 in, 2 out]
                  n427 = Write to Binary File(file (use dialog)=w914, data=w896, error in=w913, 5:w895) -> (error out=w904:errorcluster)  [unwired: 2 in, 2 out]
                  n428 = Merge Errors(w904, w903) -> (w910:errorcluster)
                }
                frame "Transfer_Settings" {
                  n429 = Unbundle By Name(w965) -> ("Device Information"=w964:string[])
                }
              }
              n430 = feedback-in #1(w806) -> ()
            }
            n431 = Release Queue(queue=w797) -> ()  [unwired: 2 in, 3 out]
          }
          frame "Measure_Spectrum" {
            w970 = T6 {"QueueAction"=enum."TimeOut", "Data"=[], "Data_Raw"=[], "Data_Dark"=[], "Data_Ref"=[], "Device Information"=[], "Numeric Control"=0.0, "Boolean"=FALSE, "Wavelength"=[], "Time"=[], "Time Stamp"=timestamp(0 s since 1904-01-01), "Numeric Control 2"=0.0, "TabControl"=enum."Measure"}  # DataQueue
            n432 = Obtain Queue(name (unnamed)="Temp", element data type=w970) -> (queue out=w969:refnum<queue>)  [unwired: 3 in, 2 out]
            n433 = while {
              shift-right: [w979] -> w973
              shift-left: w974 -> [w987]
              shift-right: [w980] -> w972
              shift-left: w975 -> [w988]
              shift-right: [w981] -> w968
              shift-left: w969 -> [w983]
              tunnel: w967 -> [w977]
              stop <- w978 stop-if-true
              n434 = Dequeue Element(queue=w987, error in (no error)=w988) -> (queue out=w985:refnum<queue>, element=w982:T6, error out=w984:errorcluster)  [unwired: 1 in, 1 out]
              n435 = Unbundle By Name(w982) -> ("QueueAction"=w986:T7, "TabControl"=w976:T8)
              n436 = case shown="\"Spectrometer_Measure\"" w986 {
                tunnel: w985 -> [w989 w1017 w1057]
                tunnel: w984 -> [w992 w1027 w1056]
                tunnel: w983 -> [w994 w1033 w1059]
                tunnel: w982 -> [w990 w1006 _]
                tunnel: [w993 w1033 w1055] -> w981
                tunnel: [w991 w1018 w1053] -> w980
                tunnel: [w989 w1017 w1054] -> w979
                tunnel: [_ _ TRUE] -> w978
                tunnel: w977 -> [_ w1010 _]
                tunnel: w976 -> [_ w1004 w1051]
                frame Default {
                  n437 = Enqueue Element(queue=w994, element=w990, error in (no error)=w992) -> (queue out=w993:refnum<queue>, error out=w991:errorcluster)  [unwired: 1 in, 1 out]
                }
                frame "Spectrometer_Measure" {
                  n438 = Unbundle By Name(w1006) -> ("Data_Raw"=w1024:T11)
                  n439 = case shown="\"Spectral Stability\"" w1004 {
                    tunnel: [w1046 "SpectralStability_SavePath"] -> w997
                    tunnel: [w1045 "SpectralStability_FileName"] -> w995
                    tunnel: [w1041 "SpectralStability_Comments"] -> w998
                    frame "Measure", Default {
                      n440 = property on="Spectra Count" class="DigNum (strict)"() -> ("Value"=w1047:u16)  [unwired: 2 in, 2 out]
                      n441 = property on="Measure_SavePath" class="Path"() -> ("Value"=w1046:path)  [unwired: 2 in, 2 out]
                      n442 = property on="Measure_Comments" class="Str"() -> ("Value"=w1041:string)  [unwired: 2 in, 2 out]
                      n443 = property on="Measure_FileName" class="Str"() -> ("Value"=w1042:string)  [unwired: 2 in, 2 out]
                      n444 = Number To Decimal String(number=w1047) -> (decimal integer string=w1043:string)  [unwired: 1 in]
                      n445 = Concatenate Strings(w1042, "_", w1043) -> (w1045:string)
                    }
                    frame "Spectral Stability" {
                    }
                  }
                  n446 = Index Array(array=w1024, index=0) -> (element=w1022:T14)
                  n447 = Unbundle By Name(w1006) -> ("Time Stamp"=w1005:timestamp)
                  n448 = Unbundle By Name(w1022) -> ("Image"=w1000:dbl[][][])
                  n449 = Index Array(array=w1000, index (dim 1)=0 ("disabled index (row)")) -> (element=w1016:dbl[][])  [unwired: 2 in]
                  n450 = Transpose 2D Array(2D array=w1016) -> (transposed array=w1013:dbl[][])
                  n451 = Format Date/Time String(time format string (%c)="%Y%m%d_%H%M%S", seconds (now)=w1005) -> (date/time string=w1031:string)  [unwired: 1 in]
                  n452 = Matrix Size(0:w1013) -> (2:w1014:i32)  [unwired: 1 out]
                  n453 = Empty String/Path?(string/path=w998) -> (empty?=w999:bool)
                  n454 = Reciprocal(x=w1014) -> (1/x=w1015:dbl)
                  n455 = Concatenate Strings(w1031, "_") -> (w996:string)
                  n456 = case shown="False" w999 {
                    tunnel: w998 -> [w1040 _]
                    tunnel: w997 -> [w1039 _]
                    tunnel: w996 -> [w1038 _]
                    tunnel: w995 -> [w1037 _]
                    frame False {
                      n457 = Concatenate Strings(w1038, w1037, "_comments.txt" ("string")) -> (w1034:string)
                      n458 = Build Path(base path=w1039, name or relative path=w1034) -> (appended path=w1035:path)
                      n459 = Write to Text File(file (use dialog)=w1035, text=w1040) -> ()  [unwired: 2 in, 3 out]
                    }
                    frame True {
                    }
                  }
                  n460 = Initialize Array(w1015, w1014) -> (w1012:dbl[])
                  n461 = Concatenate Strings(w996, w995, ".spectra" ("string")) -> (w1002:string)
                  n462 = Unbundle By Name(w1010) -> ("Wavlength"=w1007:dbl[unit][])
                  n463 = call-poly <vilib>:"A x B.vi"("Vector"=w1012, "A"=w1013) -> ("A x Vector"=w1001:dbl[])  [unwired: 1 out]
                  n464 = Build Path(base path=w997, name or relative path=w1002) -> (appended path=w1029:path)
                  n465 = Bundle("Wavlength"=w1007, "A x Vector"=w1001) -> (w1009:T15)  [unwired: 1 in]
                  n466 = Open/Create/Replace File(file path (use dialog)=w1029, error in=w1027, operation (0:open)=T13."open or create") -> (refnum out=w1026:refnum<file>, error out=w1025:errorcluster)  [unwired: 3 in, 1 out]
                  n467 = Build Array(w1009) -> (w1008:T16)
                  n468 = To Unsigned Word Integer(number=w1000) -> (unsigned 16bit integer=w1021:u16[][][])
                  n469 = property on="Measure_Graph" class="XYGraph (strict)"("Value"=w1008) -> ()  [unwired: 2 in, 2 out]
                  n470 = Write to Binary File(file (use dialog)=w1026, data=w1021, error in=w1025) -> (refnum out=w1019:refnum<file>, error out=w1020:errorcluster)  [unwired: 3 in, 1 out]
                  n471 = Close File(refnum=w1019, error in=w1020) -> (error out=w1018:errorcluster)  [unwired: 1 out]
                }
                frame "Stop_Measurement" {
                  w1052 = FALSE ("Measure Spectrum")
                  n472 = case shown="Default" w1051 {
                    frame Default {
                    }
                    frame "Measure" {
                      n473 = property on="Automatically \nadjust count" class="Bool (strict)"() -> ("Value"=w1062:bool)  [unwired: 2 in, 2 out]
                      n474 = case shown="True" w1062 {
                        frame False {
                        }
                        frame True {
                          n475 = Increment(x="Spectra Count") -> (x+1=w1063:u16)
                          n476 = property on="Spectra Count" class="DigNum (strict)"("Value"=w1063) -> ()  [unwired: 2 in, 2 out]
                        }
                      }
                    }
                  }
                  n477 = Get Queue Status(queue=w1059) -> (queue out=w1060:refnum<queue>, # elements in queue=w1058:i32)  [unwired: 2 in, 6 out]
                  n478 = property on="SpectralStability_MeasureSpectrum" class="Bool (strict)"("Value"=w1052) -> ()  [unwired: 2 in, 2 out]
                  n479 = property on="Measure_MeasureSpectrum" class="Bool (strict)"("Value"=w1052) -> ()  [unwired: 2 in, 2 out]
                  n480 = for {
                    N: w1058 -> [_]
                    shift-right: [w1070] -> w1055
                    shift-left: w1060 -> [w1071]
                    shift-right: [w1067] -> w1054
                    shift-left: w1057 -> [w1068]
                    shift-right: [w1065] -> w1053
                    shift-left: w1056 -> [w1066]
                    n481 = Dequeue Element(queue=w1071) -> (queue out=w1070:refnum<queue>, element=w1069:T6)  [unwired: 2 in, 2 out]
                    n482 = Enqueue Element(queue=w1068, element=w1069, error in (no error)=w1066) -> (queue out=w1067:refnum<queue>, error out=w1065:errorcluster)  [unwired: 1 in, 1 out]
                  }
                }
              }
            }
            n483 = Release Queue(queue=w968) -> ()  [unwired: 2 in, 3 out]
          }
          frame "Measure_SpectrumAdvanced" {
            w1075 = T6 {"QueueAction"=enum."TimeOut", "Data"=[], "Data_Raw"=[], "Data_Dark"=[], "Data_Ref"=[], "Device Information"=[], "Numeric Control"=0.0, "Boolean"=FALSE, "Wavelength"=[], "Time"=[], "Time Stamp"=timestamp(0 s since 1904-01-01), "Numeric Control 2"=0.0, "TabControl"=enum."Measure"}  # DataQueue
            n484 = Obtain Queue(name (unnamed)="Temp", element data type=w1075) -> (queue out=w1074:refnum<queue>)  [unwired: 3 in, 2 out]
            n485 = while {
              shift-right: [w1083] -> w1078
              shift-left: w1079 -> [w1091]
              shift-right: [w1084] -> w1077
              shift-left: w1080 -> [w1092]
              shift-right: [w1085] -> w1073
              shift-left: w1074 -> [w1087]
              tunnel: w1072 -> [w1081]
              stop <- w1082 stop-if-true
              n486 = Dequeue Element(queue=w1091, error in (no error)=w1092) -> (queue out=w1089:refnum<queue>, element=w1086:T6, error out=w1088:errorcluster)  [unwired: 1 in, 1 out]
              n487 = Unbundle By Name(w1086) -> ("QueueAction"=w1090:T7)
              n488 = case shown="\"Stop_Measurement\"" w1090 {
                tunnel: w1089 -> [w1093 w1117 w1143]
                tunnel: w1088 -> [w1096 w1127 w1142]
                tunnel: w1087 -> [w1098 w1136 w1145]
                tunnel: w1086 -> [w1094 w1104 _]
                tunnel: [w1097 w1136 w1141] -> w1085
                tunnel: [w1095 w1118 w1139] -> w1084
                tunnel: [w1093 w1117 w1140] -> w1083
                tunnel: [_ _ TRUE] -> w1082
                tunnel: w1081 -> [_ w1109 _]
                frame Default {
                  n489 = Enqueue Element(queue=w1098, element=w1094, error in (no error)=w1096) -> (queue out=w1097:refnum<queue>, error out=w1095:errorcluster)  [unwired: 1 in, 1 out]
                }
                frame "Spectrometer_Measure" {
                  w1133 = "_"
                  n490 = Unbundle By Name(w1104) -> ("Time Stamp"=w1103:timestamp)
                  n491 = property on="Nr After Spin" class="DigNum (strict)"() -> ("Value"=w1102:u16)  [unwired: 2 in, 2 out]
                  n492 = Unbundle By Name(w1109) -> ("Wavlength"=w1106:dbl[unit][])
                  n493 = property on="Measure_FileName" class="Str"() -> ("Value"=w1132:string)  [unwired: 2 in, 2 out]
                  n494 = Number To Decimal String(number=w1102) -> (decimal integer string=w1100:string)  [unwired: 1 in]
                  n495 = Format Date/Time String(time format string (%c)="%Y%m%d_%H%M%S", seconds (now)=w1103) -> (date/time string=w1134:string)  [unwired: 1 in]
                  n496 = Concatenate Strings(w1134, w1133, w1132, w1133, "a" ("string"), w1100, ".spectra" ("string")) -> (w1131:string)
                  n497 = property on="Measure_SavePath" class="Path"() -> ("Value"=w1130:path)  [unwired: 2 in, 2 out]
                  n498 = Build Path(base path=w1130, name or relative path=w1131) -> (appended path=w1129:path)
                  n499 = Unbundle By Name(w1104) -> ("Data_Raw"=w1124:T11)
                  n500 = Open/Create/Replace File(file path (use dialog)=w1129, error in=w1127, operation (0:open)=T13."open or create") -> (refnum out=w1126:refnum<file>, error out=w1125:errorcluster)  [unwired: 3 in, 1 out]
                  n501 = Index Array(array=w1124, index=0) -> (element=w1122:T14)
                  n502 = Unbundle By Name(w1122) -> ("Image"=w1110:dbl[][][])
                  n503 = Index Array(array=w1110, index (dim 1)=0 ("disabled index (row)")) -> (element=w1116:dbl[][])  [unwired: 2 in]
                  n504 = Transpose 2D Array(2D array=w1116) -> (transposed array=w1113:dbl[][])
                  n505 = To Unsigned Word Integer(number=w1110) -> (unsigned 16bit integer=w1121:u16[][][])
                  n506 = Matrix Size(0:w1113) -> (2:w1114:i32)  [unwired: 1 out]
                  n507 = Write to Binary File(file (use dialog)=w1126, data=w1121, error in=w1125) -> (refnum out=w1119:refnum<file>, error out=w1120:errorcluster)  [unwired: 3 in, 1 out]
                  n508 = Reciprocal(x=w1114) -> (1/x=w1115:dbl)
                  n509 = Close File(refnum=w1119, error in=w1120) -> (error out=w1118:errorcluster)  [unwired: 1 out]
                  n510 = Initialize Array(w1115, w1114) -> (w1112:dbl[])
                  n511 = call-poly <vilib>:"A x B.vi"("Vector"=w1112, "A"=w1113) -> ("A x Vector"=w1105:dbl[])  [unwired: 1 out]
                  n512 = Bundle("Wavlength"=w1106, "A x Vector"=w1105) -> (w1108:T15)  [unwired: 1 in]
                  n513 = Build Array(w1108) -> (w1107:T16)
                  n514 = property on="Measure_Graph" class="XYGraph (strict)"("Value"=w1107) -> ()  [unwired: 2 in, 2 out]
                }
                frame "Stop_Measurement" {
                  n515 = property on="Automatically \nadjust count" class="Bool (strict)"() -> ("Value"=w1137:bool)  [unwired: 2 in, 2 out]
                  n516 = case shown="True" w1137 {
                    frame False {
                    }
                    frame True {
                      n517 = property on="Nr After Spin" class="DigNum (strict)"() -> ("Value"=w1149:u16)  [unwired: 2 in, 2 out]
                      n518 = Increment(x=w1149) -> (x+1=w1148:u16)
                      n519 = property on="Nr After Spin" class="DigNum (strict)"("Value"=w1148) -> ()  [unwired: 2 in, 2 out]
                    }
                  }
                  n520 = Get Queue Status(queue=w1145) -> (queue out=w1146:refnum<queue>, # elements in queue=w1144:i32)  [unwired: 2 in, 6 out]
                  n521 = property on="Measure_MeasureSpectrum" class="Bool (strict)"("Value"=FALSE ("Measure Spectrum")) -> ()  [unwired: 2 in, 2 out]
                  n522 = for {
                    N: w1144 -> [_]
                    shift-right: [w1155] -> w1141
                    shift-left: w1146 -> [w1156]
                    shift-right: [w1152] -> w1140
                    shift-left: w1143 -> [w1153]
                    shift-right: [w1150] -> w1139
                    shift-left: w1142 -> [w1151]
                    n523 = Dequeue Element(queue=w1156) -> (queue out=w1155:refnum<queue>, element=w1154:T6)  [unwired: 2 in, 2 out]
                    n524 = Enqueue Element(queue=w1153, element=w1154, error in (no error)=w1151) -> (queue out=w1152:refnum<queue>, error out=w1150:errorcluster)  [unwired: 1 in, 1 out]
                  }
                }
              }
            }
            n525 = Release Queue(queue=w1073) -> ()  [unwired: 2 in, 3 out]
          }
          frame "Measure_SpectralStability" {
            w1172 = T6 {"QueueAction"=enum."TimeOut", "Data"=[], "Data_Raw"=[], "Data_Dark"=[], "Data_Ref"=[], "Device Information"=[], "Numeric Control"=0.0, "Boolean"=FALSE, "Wavelength"=[], "Time"=[], "Time Stamp"=timestamp(0 s since 1904-01-01), "Numeric Control 2"=0.0, "TabControl"=enum."Measure"}  # DataQueue
            n526 = Unbundle By Name(w1161) -> ("Time Stamp"=w1167:timestamp)
            n527 = Unbundle By Name(w1161) -> ("Numeric Control"=w1157:dbl)
            n528 = property on="SpectralStability\n_SavePath" class="Path"() -> ("Value"=w1163:path)  [unwired: 2 in, 2 out]
            n529 = property on="SpectralStability\n_FileName" class="Str"() -> ("Value"=w1162:string)  [unwired: 2 in, 2 out]
            n530 = Obtain Queue(name (unnamed)="Temp", element data type=w1172) -> (queue out=w1171:refnum<queue>)  [unwired: 3 in, 2 out]
            n531 = call "Num2Str_TrailingZero.vi"("Numeric Control"=w1157) -> ("format string"=w1160:string)  [unwired: 10 in]
            n532 = Format Date/Time String(time format string (%c)="%Y%m%d_%H%M%S", seconds (now)=w1167) -> (date/time string=w1164:string)  [unwired: 1 in]
            n533 = while {
              shift-right: [w1177] -> w1165
              shift-left: w1174 -> [w1177]
              shift-right: [w1183] -> _
              shift-left: w1171 -> [w1185]
              border: 0 -> [_]
              shift-right: [w1184] -> w1158
              shift-left: w1169 -> [w1193]
              shift-right: [w1182] -> w1159
              shift-left: w1168 -> [w1192]
              tunnel: w1164 -> [w1180]
              tunnel: w1163 -> [w1179]
              tunnel: w1162 -> [w1178]
              tunnel: w1160 -> [w1176]
              tunnel: w1157 -> [w1175]
              stop <- w1181 stop-if-true
              n534 = Dequeue Element(queue=w1193, error in (no error)=w1192) -> (queue out=w1191:refnum<queue>, element=w1189:T6, error out=w1190:errorcluster)  [unwired: 1 in, 1 out]
              n535 = Unbundle By Name(w1189) -> ("QueueAction"=w1188:T7)
              n536 = feedback #2() -> (w1186:i32)
              n537 = case shown="\"Spectrometer_Measure\"" w1188 {
                tunnel: w1191 -> [w1197 w1206 w1212 w1230 w1313 w1320]
                tunnel: w1190 -> [w1196 w1203 w1213 w1231 _ w1321]
                tunnel: w1189 -> [w1198 w1202 _ _ w1267 w1352]
                tunnel: [w1200 w1208 w1219 w1237 w1251 w1353] -> w1187
                tunnel: w1186 -> [w1200 w1208 w1219 w1237 w1311 w1353]
                tunnel: w1185 -> [w1199 w1207 w1215 w1233 w1312 w1330]
                tunnel: [w1197 w1205 w1210 w1228 w1313 w1320] -> w1184
                tunnel: [w1195 w1207 w1214 w1232 w1312 w1330] -> w1183
                tunnel: [w1194 w1204 w1211 w1229 w1256 w1321] -> w1182
                tunnel: [_ TRUE TRUE TRUE _ _] -> w1181
                tunnel: w1180 -> [_ _ _ _ w1309 w1350]
                tunnel: w1179 -> [_ _ _ _ w1276 w1318]
                tunnel: w1178 -> [_ _ _ _ w1308 w1348]
                tunnel: w1177 -> [_ _ _ _ w1283 w1347]
                tunnel: w1176 -> [_ _ _ _ w1310 _]
                tunnel: w1175 -> [_ _ _ _ w1252 _]
                frame Default {
                  n538 = Enqueue Element(queue=w1199, element=w1198, error in (no error)=w1196) -> (queue out=w1195:refnum<queue>, error out=w1194:errorcluster)  [unwired: 1 in, 1 out]
                }
                frame "Close_Program" {
                  n539 = Enqueue Element At Opposite End(queue=w1206, element=w1202, error in (no error)=w1203) -> (queue out=w1205:refnum<queue>, error out=w1204:errorcluster)  [unwired: 1 in, 1 out]
                }
                frame "Abort" {
                  n540 = Get Queue Status(queue=w1215) -> (queue out=w1217:refnum<queue>, # elements in queue=w1218:i32)  [unwired: 2 in, 6 out]
                  n541 = for {
                    N: w1218 -> [_]
                    shift-right: [w1225] -> w1214
                    shift-left: w1217 -> [w1226]
                    shift-right: [w1222] -> w1210
                    shift-left: w1212 -> [w1223]
                    shift-right: [w1220] -> w1211
                    shift-left: w1213 -> [w1221]
                    n542 = Dequeue Element(queue=w1226) -> (queue out=w1225:refnum<queue>, element=w1224:T6)  [unwired: 2 in, 2 out]
                    n543 = Enqueue Element(queue=w1223, element=w1224, error in (no error)=w1221) -> (queue out=w1222:refnum<queue>, error out=w1220:errorcluster)  [unwired: 1 in, 1 out]
                  }
                  n544 = property on="SpectralStability_Record" class="Bool (strict)"("Value"=FALSE ("SpectralStability_Record")) -> ()  [unwired: 2 in, 2 out]
                }
                frame "Stop_Measurement" {
                  n545 = Get Queue Status(queue=w1233) -> (queue out=w1235:refnum<queue>, # elements in queue=w1236:i32)  [unwired: 2 in, 6 out]
                  n546 = for {
                    N: w1236 -> [_]
                    shift-right: [w1243] -> w1232
                    shift-left: w1235 -> [w1244]
                    shift-right: [w1240] -> w1228
                    shift-left: w1230 -> [w1241]
                    shift-right: [w1238] -> w1229
                    shift-left: w1231 -> [w1239]
                    n547 = Dequeue Element(queue=w1244) -> (queue out=w1243:refnum<queue>, element=w1242:T6)  [unwired: 2 in, 2 out]
                    n548 = Enqueue Element(queue=w1241, element=w1242, error in (no error)=w1239) -> (queue out=w1240:refnum<queue>, error out=w1238:errorcluster)  [unwired: 1 in, 1 out]
                  }
                  n549 = property on="SpectralStability_Record" class="Bool (strict)"("Value"=FALSE ("SpectralStability_Record")) -> ()  [unwired: 2 in, 2 out]
                }
                frame "Spectrometer_Measure" {
                  w1307 = "_"
                  n550 = Increment(x=w1311) -> (x+1=w1251:i32)
                  n551 = Unbundle By Name(w1267) -> ("Numeric Control 2"=w1266:dbl)
                  n552 = Unbundle By Name(w1267) -> ("Data_Raw"=w1305:T11)
                  n553 = Format Into String(format string=w1310, w1311) -> (resulting string=w1265:string)  [unwired: 2 in, 1 out]
                  n554 = Concatenate Strings(w1309, w1307, w1308, w1307) -> (w1278:string)
                  n555 = Unbundle By Name(w1283) -> ("Wavlength"=w1281:dbl[unit][])
                  n556 = Index Array(array=w1305, index=0) -> (element=w1303:T14)
                  n557 = Divide(x=w1251, y=w1252) -> (x/y=w1255:dbl)
                  n558 = Concatenate Strings(w1278, "s" ("string"), w1265, ".smean" ("string")) -> (w1287:string)
                  n559 = Concatenate Strings(w1278, "raw" ("string"), w1265, ".spectra" ("string")) -> (w1295:string)
                  n560 = Unbundle By Name(w1303) -> ("Image"=w1291:dbl[][][])
                  n561 = Concatenate Strings(w1278, "timing.txt" ("string")) -> (w1275:string)
                  n562 = Subtract(x=w1252, y=w1251) -> (x-y=w1247:dbl)
                  "SS_StepsLeft" <- w1247
                  n563 = Number To Exponential String(number=w1266, 1:FALSE ("use system decimal point (T)")) -> (E-format string=w1263:string)  [unwired: 2 in]
                  n564 = Build Path(base path=w1276, name or relative path=w1287) -> (appended path=w1284:path)
                  n565 = Build Path(base path=w1276, name or relative path=w1275) -> (appended path=w1274:path)
                  n566 = Multiply(x=w1255, y=100.0) -> (x*y=w1254:dbl)
                  n567 = property on="SS:PeriodicTime" class="DigNum (strict)"() -> ("Value"=w1249:dbl[unit])  [unwired: 2 in, 2 out]
                  n568 = Build Path(base path=w1276, name or relative path=w1295) -> (appended path=w1292:path)
                  n569 = Index Array(array=w1291, index (dim 1)=0 ("disabled index (row)")) -> (element=w1302:dbl[][])  [unwired: 2 in]
                  n570 = To Unsigned Byte Integer(number=w1254) -> (unsigned 8bit integer=→"Horizontal Progress Bar":u8)
                  n571 = To Unsigned Word Integer(number=w1291) -> (unsigned 16bit integer=w1290:u16[][][])
                  n572 = Open/Create/Replace File(file path (use dialog)=w1274, operation (0:open)=T13."open or create") -> (refnum out=w1272:refnum<file>, error out=w1269:errorcluster)  [unwired: 4 in, 1 out]
                  n573 = Concatenate Strings(w1265, "\t", w1263, "\r\n") -> (w1262:string)
                  n574 = Transpose 2D Array(2D array=w1302) -> (transposed array=w1299:dbl[][])
                  n575 = Write to Binary File(file (use dialog)=w1292, data=w1290) -> (refnum out=w1288:refnum<file>, error out=w1289:errorcluster)  [unwired: 4 in, 1 out]
                  n576 = Multiply(x=w1249, y=w1247) -> (x*y=→"SS_TimePrediction":dbl[unit])
                  n577 = Set File Position(refnum=w1272, from (0:start)=enum16{"start", "end", "current"}."end", error in=w1269) -> (refnum out=w1270:refnum<file>, error out=w1268:errorcluster)  [unwired: 1 in]
                  n578 = Matrix Size(0:w1299) -> (2:w1300:i32)  [unwired: 1 out]
                  n579 = Close File(refnum=w1288, error in=w1289) -> (error out=w1259:errorcluster)  [unwired: 1 out]
                  n580 = Reciprocal(x=w1300) -> (1/x=w1301:dbl)
                  n581 = Write to Text File(file (use dialog)=w1270, text=w1262, error in=w1268) -> (refnum out=w1261:refnum<file>, error out=w1260:errorcluster)  [unwired: 1 in, 1 out]
                  n582 = Initialize Array(w1301, w1300) -> (w1298:dbl[])
                  n583 = call-poly <vilib>:"A x B.vi"("Vector"=w1298, "A"=w1299) -> ("A x Vector"=w1280:dbl[])  [unwired: 1 out]
                  n584 = Bundle("Wavlength"=w1281, "A x Vector"=w1280) -> (w1282:T15)  [unwired: 1 in]
                  n585 = Close File(refnum=w1261, error in=w1260) -> (error out=w1257:errorcluster)  [unwired: 1 out]
                  n586 = Write to Binary File(file (use dialog)=w1284, data=w1280) -> (refnum out=w1286:refnum<file>, error out=w1285:errorcluster)  [unwired: 4 in, 1 out]
                  n587 = Build Array(w1282) -> (w1279:T16)
                  n588 = Close File(refnum=w1286, error in=w1285) -> (error out=w1258:errorcluster)  [unwired: 1 out]
                  n589 = property on="SpectralStability:\nGraph" class="XYGraph (strict)"("Value"=w1279) -> ()  [unwired: 2 in, 2 out]
                  n590 = Merge Errors(w1259, w1258, w1257) -> (w1256:errorcluster)
                }
                frame "Transfer_Settings" {
                  w1323 = "\r\n"
                  w1337 = 0.0
                  w1343 = 0 ("index")
                  n591 = Unbundle By Name(w1347) -> ("Dark"=w1344:T11, "Ref"=w1345:T11, "Wavlength"=w1346:dbl[unit][])
                  n592 = Concatenate Strings(w1350, "_", w1348) -> (w1336:string)
                  n593 = property on="SpectralStability_\nPeriodicTime" class="DigNum (strict)"() -> ("Value"=w1329:dbl[unit])  [unwired: 2 in, 2 out]
                  n594 = Unbundle By Name(w1352) -> ("Device Information"=w1351:string[])
                  n595 = property on="SpectralStability_Duration" class="DigNum (strict)"() -> ("Value"=w1328:dbl[unit])  [unwired: 2 in, 2 out]
                  n596 = Index Array(array=w1344, index=w1343) -> (element=w1341:T14)
                  n597 = Index Array(array=w1345, index=w1343) -> (element=w1342:T14)
                  n598 = Concatenate Strings(w1336, "_add.spin" ("string")) -> (w1333:string)
                  n599 = Concatenate Strings(w1336, "_comments.txt" ("string")) -> (w1319:string)
                  n600 = Unbundle By Name(w1341) -> ("Image"=w1315:dbl[][][])
                  n601 = Unbundle By Name(w1342) -> ("Image"=w1314:dbl[][][])
                  n602 = property on="SpectralStability_\nMeasurementNumber" class="DigNum (strict)"() -> ("Value"=w1327:u32)  [unwired: 2 in, 2 out]
                  n603 = Build Path(base path=w1318, name or relative path=w1333) -> (appended path=w1332:path)
                  n604 = Build Path(base path=w1318, name or relative path=w1319) -> (appended path=w1317:path)
                  n605 = node(w1346) -> (w1338:dbl[])
                  n606 = property on="Duration/Times" class="Bool (strict)"() -> ("Value"=w1326:bool)  [unwired: 2 in, 2 out]
                  n607 = To Unsigned Word Integer(number=w1315) -> (unsigned 16bit integer=w1340:u16[][][])
                  n608 = To Unsigned Word Integer(number=w1314) -> (unsigned 16bit integer=w1339:u16[][][])
                  n609 = call "DeviceInfo2Str.vi"("Device Information"=w1351) -> ("String"=w1325:string)  [unwired: 10 in]
                  n610 = property on="SpectralStability:\nComments" class="Str"() -> ("Value"=w1322:string)  [unwired: 2 in, 2 out]
                  n611 = Bundle(w1340, w1339, w1338, w1337, w1337) -> (w1331:cluster{u16[][][], u16[][][], dbl[], dbl, dbl})  [unwired: 1 in]
                  n612 = call "String_SpectralStabilitySettings.vi"("Duration/Times"=w1326, "Measurement Number"=w1327, "Duration"=w1328, "Periodic Time"=w1329) -> ("String"=w1324:string)  [unwired: 7 in]
                  n613 = Concatenate Strings(w1325, w1323, w1324, w1323, w1322) -> (w1316:string)
                  n614 = Write to Binary File(file (use dialog)=w1332, data=w1331) -> ()  [unwired: 4 in, 3 out]
                  n615 = Write to Text File(file (use dialog)=w1317, text=w1316) -> ()  [unwired: 2 in, 3 out]
                }
              }
              n616 = feedback-in #2(w1187) -> ()
            }
          }
          frame "Save_InSitu" {
            w1357 = "\r\n"
            n617 = Unbundle By Name(w1395) -> ("Time Stamp"=w1393:timestamp, "Device Information"=w1384:string[], "Numeric Control"=w1381:dbl, "Numeric Control 2"=w1380:dbl)
            n618 = Unbundle By Name(w1382) -> ("Dark"=w1401:T11, "Ref"=w1399:T11, "Wavlength"=w1403:dbl[unit][])
            n619 = node(w1403) -> (w1396:dbl[])
            n620 = property on="Frames" class="DigNum (strict)"() -> ("Value"=w1368:i32)  [unwired: 2 in, 2 out]
            n621 = call "DeviceInfo2Str.vi"("Device Information"=w1384) -> ("String"=w1383:string)  [unwired: 10 in]
            n622 = Number To Decimal String(number=w1368) -> (decimal integer string=w1367:string)  [unwired: 1 in]
            n623 = property on="Seconds after Spin" class="DigNum (strict)"() -> ("Value"=w1364:dbl[unit])  [unwired: 2 in, 2 out]
            n624 = property on="Seconds to Spin" class="DigNum (strict)"() -> ("Value"=w1365:dbl[unit])  [unwired: 2 in, 2 out]
            n625 = Index Array(array=w1399, index=0) -> (element=w1397:T14)
            n626 = Index Array(array=w1401, index=0) -> (element=w1398:T14)
            n627 = property on="Measure_FileName" class="Str"() -> ("Value"=w1377:string)  [unwired: 2 in, 2 out]
            n628 = property on="Program Spin Coater" class="Arr (strict)"() -> ("Value"=w1366:T2)  [unwired: 2 in, 2 out]
            n629 = Unbundle By Name(w1398) -> ("Image"=w1354:dbl[][][])
            n630 = Unbundle By Name(w1397) -> ("Image"=w1355:dbl[][][])
            n631 = Format Date/Time String(time format string (%c)="%Y%m%d_%H%M%S", seconds (now)=w1393) -> (date/time string=w1392:string)  [unwired: 1 in]
            n632 = call "MeasurementSpin2String.vi"("Seconds after Spin Stop"=w1364, "Seconds to Spin Start"=w1365, "Program Spin Coater"=w1366) -> ("concatenated string"=w1363:string)
            n633 = property on="Duration after" class="DigNum (strict)"() -> ("Value"=w1360:dbl[unit])  [unwired: 2 in, 2 out]
            n634 = Concatenate Strings(w1392, "_" ("string"), w1377) -> (w1390:string)
            n635 = property on="periodic time" class="DigNum (strict)"() -> ("Value"=w1361:dbl[unit])  [unwired: 2 in, 2 out]
            n636 = To Unsigned Word Integer(number=w1354) -> (unsigned 16bit integer=w1371:u16[][][])
            n637 = property on="Spin at end" class="Bool (strict)"() -> ("Value"=w1359:bool)  [unwired: 2 in, 2 out]
            n638 = To Unsigned Word Integer(number=w1355) -> (unsigned 16bit integer=w1370:u16[][][])
            n639 = call "AfterSpinOptions.vi"("Spin at end"=w1359, "Duration after"=w1360, "periodic time"=w1361) -> ("concatenated string"=w1362:string)  [unwired: 8 in]
            n640 = Concatenate Strings(w1383, w1357, "Frames:\t" ("string"), w1367, w1357, w1363, w1357, w1362, w1357, "Comments:" ("string"), w1357, "Measure_Comments") -> (w1379:string)
            n641 = Bundle(w1371, w1370, w1396, "Numeric Control"=w1381, "Numeric Control 2"=w1380) -> (w1374:T17)  [unwired: 1 in]
            n642 = property on="Measure_SavePath" class="Path"() -> ("Value"=w1376:path)  [unwired: 2 in, 2 out]
            n643 = Concatenate Strings(w1390, "_add.spin" ("string")) -> (w1388:string)
            n644 = Concatenate Strings(w1390, "_comments.txt" ("string")) -> (w1387:string)
            n645 = Build Path(base path=w1376, name or relative path=w1388) -> (appended path=w1375:path)
            n646 = Build Path(base path=w1376, name or relative path=w1387) -> (appended path=w1386:path)
            n647 = Write to Text File(file (use dialog)=w1386, text=w1379) -> (error out=w1373:errorcluster)  [unwired: 2 in, 2 out]
            n648 = Write to Binary File(file (use dialog)=w1375, data=w1374) -> (error out=w1372:errorcluster)  [unwired: 4 in, 2 out]
            n649 = flat-sequence {
              tunnel: w1373 -> [_]
              tunnel: w1372 -> [_]
              frame #0 {
                n650 = property on="Action" class="Str"("Value"="" ("Action")) -> ()  [unwired: 2 in, 2 out]
              }
            }
            n651 = property on="Action" class="Str"("Value"="Saving" ("Action")) -> ()  [unwired: 2 in, 2 out]
          }
          frame "Set_Dark" {
            # "Averaging"
            n652 = Unbundle By Name(w1418) -> ("Wavlength"=w1417:dbl[unit][])
            n653 = Unbundle By Name(w1425) -> ("Data_Dark"=w1415:T11)
            n654 = Index Array(array=w1415, index=0) -> (element=w1420:T14)
            n655 = Unbundle By Name(w1420) -> ("Image"=w1414:dbl[][][])
            n656 = Index Array(array=w1414, index (dim 1)=0 ("disabled index (row)")) -> (element=w1412:dbl[][])  [unwired: 2 in]
            n657 = Transpose 2D Array(2D array=w1412) -> (transposed array=w1409:dbl[][])
            n658 = Matrix Size(0:w1409) -> (2:w1410:i32)  [unwired: 1 out]
            n659 = Reciprocal(x=w1410) -> (1/x=w1411:dbl)
            n660 = Initialize Array(w1411, w1410) -> (w1408:dbl[])
            n661 = call-poly <vilib>:"A x B.vi"("Vector"=w1408, "A"=w1409) -> ("A x Vector"=w1407:dbl[])  [unwired: 1 out]
            n662 = Bundle("Wavlength"=w1417, "A x Vector"=w1407) -> (w1419:T15)  [unwired: 1 in]
            n663 = Build Array(w1419) -> (w1416:T16)
            n664 = property on="Measure_Graph" class="XYGraph (strict)"("Value"=w1416) -> ()  [unwired: 2 in, 2 out]
            n665 = Bundle By Name(cluster=w1418, "Dark"=w1415) -> (w1422:T4)
          }
          frame "Set_Ref" {
            # "Averaging"
            n666 = Unbundle By Name(w1427) -> ("Wavlength"=w1426:dbl[unit][])
            n667 = Unbundle By Name(w1444) -> ("Data_Ref"=w1431:T11)
            n668 = Index Array(array=w1431, index=0) -> (element=w1439:T14)
            n669 = Unbundle By Name(w1439) -> ("Image"=w1438:dbl[][][])
            n670 = Index Array(array=w1438, index (dim 1)=0 ("disabled index (row)")) -> (element=w1436:dbl[][])  [unwired: 2 in]
            n671 = Transpose 2D Array(2D array=w1436) -> (transposed array=w1433:dbl[][])
            n672 = Matrix Size(0:w1433) -> (2:w1434:i32)  [unwired: 1 out]
            n673 = Reciprocal(x=w1434) -> (1/x=w1435:dbl)
            n674 = Initialize Array(w1435, w1434) -> (w1432:dbl[])
            n675 = call-poly <vilib>:"A x B.vi"("Vector"=w1432, "A"=w1433) -> ("A x Vector"=w1428:dbl[])  [unwired: 1 out]
            n676 = Bundle("Wavlength"=w1426, "A x Vector"=w1428) -> (w1430:T15)  [unwired: 1 in]
            n677 = Build Array(w1430) -> (w1429:T16)
            n678 = Bundle By Name(cluster=w1427, "Ref"=w1431) -> (w1441:T4)
            n679 = property on="Measure_Graph" class="XYGraph (strict)"("Value"=w1429) -> ()  [unwired: 2 in, 2 out]
          }
          frame "Set_Wavelength" {
            n680 = Unbundle By Name(w1447) -> ("Wavelength"=w1450:dbl[unit][])
            n681 = Bundle By Name(cluster=w1449, "Wavlength"=w1450) -> (w1448:T4)
          }
          frame "Spectrometer_Preview" {
            w1457 = 0 ("index (page)")
            n682 = Unbundle By Name(w1453) -> ("Data_Raw"=w1461:T11)
            n683 = Unbundle By Name(w1462) -> ("Wavlength"=w1456:dbl[unit][])
            n684 = Unbundle By Name(w1453) -> ("TabControl"=w1452:T8)
            n685 = Index Array(array=w1461, index=0) -> (element=w1459:T14)
            n686 = Unbundle By Name(w1459) -> ("Image"=w1458:dbl[][][])
            n687 = Index Array(array=w1458, index (dim 0)=w1457, index (dim 1)=w1457) -> (element=w1455:dbl[])  [unwired: 1 in]
            n688 = Bundle("Wavlength"=w1456, "Image"=w1455) -> (w1454:cluster{"Wavlength":dbl[unit][], "Image":dbl[]})  [unwired: 1 in]
            n689 = Build Array(w1454) -> (w1451:T3)
            n690 = case shown="Default" w1452 {
              tunnel: w1451 -> [w1465 w1466 _]
              frame "Measure" {
                "Measure_Graph" <- w1465
              }
              frame "Spectral Stability" {
                "SpectralStability_Graph" <- w1466
              }
              frame Default {
              }
            }
          }
        }
      }
      frame Error {
        w1472 = T12 4 items=["no dialog", "OK message", "continue or stop message", "OK message + warnings", "continue/stop + warnings"] ("type of dialog (OK msg:1)")
        n691 = call <vilib>:"General Error Handler.vi"("type of dialog (OK msg:1)"=w1472, "error in (no error)"=w1469) -> ("error out"=w1471:errorcluster)  [unwired: 9 in, 4 out]
        n692 = call <vilib>:"Clear Errors.vi"("error in (no error)"=w1471) -> ("error out"=w1468:errorcluster)  [unwired: 5 in, 1 out]
      }
    }
  }
  n693 = while {
    shift-right: [w1475] -> _
    shift-left: w12 -> [w1473]
    shift-right: [w1478] -> _
    shift-left: w7 -> [w1479]
    shift-right: [w1476] -> _
    shift-left: w8 -> [w1477]
    stop <- w1474 stop-if-true
    # "Producer"
    n694 = event shown="[20] \"SpectralStability_Record\": Value Change" {
      selector: _ -> [_ _ _ _ _ _ _ _ _ _ _ _ _ _ _ _ _ _ _ _ _ _ _ _]
      dyn-events: _ -> [_ _ _ _ _ _ _ _ _ _ _ _ _ _ _ _ _ _ _ _ _ _ _ _]
      timeout: -1 -> [_ _ _ _ _ _ _ _ _ _ _ _ _ _ _ _ _ _ _ _ _ _ _ _]
      tunnel: w1479 -> [w1482 w1497 w1505 w1518 w1532 w1547 w1561 w1585 w1588 w1595 w1614 w1622 w1638 w1646 w1661 w1671 w1680 w1688 w1694 w1703 w1718 w1735 w1741 w1756]
      tunnel: [w1482 w1494 w1504 w1518 w1532 w1547 w1561 w1585 w1588 w1595 w1614 w1622 w1638 w1645 w1661 w1671 w1680 w1688 w1694 w1701 w1716 w1735 w1741 w1756] -> w1478
      tunnel: w1477 -> [w1481 w1496 w1508 w1516 w1529 w1546 w1559 w1580 w1587 w1592 w1612 w1621 w1636 w1652 w1658 w1670 w1679 w1687 w1693 w1707 w1722 w1736 w1740 w1754]
      tunnel: [w1481 w1490 w1499 w1512 w1528 w1544 w1557 w1579 w1587 w1590 w1611 w1619 w1635 w1644 w1659 w1667 w1676 w1687 w1693 w1707 w1722 w1736 w1740 w1751] -> w1476
      tunnel: w1473 -> [w1483 w1498 w1509 w1517 w1531 w1548 w1560 w1582 w1589 w1593 w1615 w1623 w1639 w1654 w1662 w1672 w1681 w1689 w1695 w1708 w1723 w1734 w1742 w1755]
      tunnel: [w1483 w1495 w1507 w1513 w1530 w1545 w1558 w1581 w1589 w1594 w1613 w1620 w1637 w1653 w1660 w1668 w1677 w1689 w1692 w1706 w1721 w1734 w1742 w1752] -> w1475
      tunnel: [_ TRUE _ _ _ _ _ _ _ _ _ _ _ _ _ _ _ _ _ _ _ _ _ _] -> w1474
      event Timeout {
        n695 = event-data() -> ()  [unwired: 1 in, 3 out]
      }
      event "Stop Button": Value Change {
        w1486 = T6 {"QueueAction"=enum."TimeOut", "Data"=[], "Data_Raw"=[], "Data_Dark"=[], "Data_Ref"=[], "Device Information"=[], "Numeric Control"=0.0, "Boolean"=FALSE, "Wavelength"=[], "Time"=[], "Time Stamp"=timestamp(0 s since 1904-01-01), "Numeric Control 2"=0.0, "TabControl"=enum."Measure"}  # DataQueue
        w1489 = T9 {"QueueAction"=enum."TimeOut", "Numeric 1"=0.0, "Numeric 2"=0.0, "Boolean 1"=FALSE, "Boolean 2"=FALSE, "Spin Program"=[], "Spin Prg v07"=[], "Time Stamp"=timestamp(0 s since 1904-01-01), "TabControl"=enum."Measure"}  # Device Queue
        n696 = event-data() -> ()  [unwired: 1 in, 6 out]
        n697 = Bundle By Name(cluster=w1489, "QueueAction"=DeviceQueue_Action."Close_Program") -> (w1487:T9)
        n698 = Enqueue Element At Opposite End(queue=w1498, element=w1487, error in (no error)=w1496) -> (queue out=w1495:refnum<queue>, error out=w1491:errorcluster)  [unwired: 1 in, 1 out]
        n699 = Bundle By Name(cluster=w1486, "QueueAction"=DataQueue_Action."Close_Program") -> (w1484:T6)
        n700 = Enqueue Element At Opposite End(queue=w1497, element=w1484, error in (no error)=w1496) -> (queue out=w1494:refnum<queue>, error out=w1492:errorcluster)  [unwired: 1 in, 1 out]
        n701 = Merge Errors(w1492, w1491) -> (w1490:errorcluster)
      }
      event "Abort Button": Value Change {
        w1503 = T6 {"QueueAction"=enum."TimeOut", "Data"=[], "Data_Raw"=[], "Data_Dark"=[], "Data_Ref"=[], "Device Information"=[], "Numeric Control"=0.0, "Boolean"=FALSE, "Wavelength"=[], "Time"=[], "Time Stamp"=timestamp(0 s since 1904-01-01), "Numeric Control 2"=0.0, "TabControl"=enum."Measure"}  # DataQueue
        w1511 = T9 {"QueueAction"=enum."TimeOut", "Numeric 1"=0.0, "Numeric 2"=0.0, "Boolean 1"=FALSE, "Boolean 2"=FALSE, "Spin Program"=[], "Spin Prg v07"=[], "Time Stamp"=timestamp(0 s since 1904-01-01), "TabControl"=enum."Measure"}  # Device Queue
        n702 = event-data() -> ()  [unwired: 1 in, 6 out]
        n703 = Bundle By Name(cluster=w1511, "QueueAction"=DeviceQueue_Action."Abort") -> (w1510:T9)
        n704 = Bundle By Name(cluster=w1503, "QueueAction"=DataQueue_Action."Abort") -> (w1501:T6)
        n705 = Enqueue Element At Opposite End(queue=w1509, element=w1510, error in (no error)=w1508) -> (queue out=w1507:refnum<queue>, error out=w1500:errorcluster)  [unwired: 1 in, 1 out]
        n706 = Enqueue Element At Opposite End(queue=w1505, element=w1501, error in (no error)=w1500) -> (queue out=w1504:refnum<queue>, error out=w1499:errorcluster)  [unwired: 1 in, 1 out]
      }
      event "Init_Spectrometer": Value Change {
        n707 = event-data() -> ()  [unwired: 1 in, 6 out]
        n708 = case shown="True" "Init_Spectrometer" {
          tunnel: [w1520 w1523] -> w1514
          frame True {
            n709 = property on="Tab Control" class="TabCtl (strict)"() -> ("Value"=w1519:T1)  [unwired: 2 in, 2 out]
            n710 = Bundle By Name(cluster=T9 {"QueueAction"=enum."TimeOut", "Numeric 1"=0.0, "Numeric 2"=0.0, "Boolean 1"=FALSE, "Boolean 2"=FALSE, "Spin Program"=[], "Spin Prg v07"=[], "Time Stamp"=timestamp(0 s since 1904-01-01), "TabControl"=enum."Measure"} ("element"), "QueueAction"=DeviceQueue_Action."Spectrometer_Init", "TabControl"=w1519) -> (w1520:T9)
          }
          frame False {
            n711 = Bundle By Name(cluster=T9 {"QueueAction"=enum."TimeOut", "Numeric 1"=0.0, "Numeric 2"=0.0, "Boolean 1"=FALSE, "Boolean 2"=FALSE, "Spin Program"=[], "Spin Prg v07"=[], "Time Stamp"=timestamp(0 s since 1904-01-01), "TabControl"=enum."Measure"} ("element"), "QueueAction"=DeviceQueue_Action."Spectrometer_Close") -> (w1523:T9)
          }
        }
        n712 = Enqueue Element(queue=w1517, element=w1514, error in (no error)=w1516) -> (queue out=w1513:refnum<queue>, error out=w1512:errorcluster)  [unwired: 1 in, 1 out]
      }
      event "Init_Arduino": Value Change {
        n713 = event-data() -> ("NewVal"=w1527:bool)  [unwired: 1 in, 5 out]
        n714 = case shown="True" w1527 {
          tunnel: [w1533 w1536] -> w1526
          frame False {
            w1535 = T9 {"QueueAction"=enum."TimeOut", "Numeric 1"=0.0, "Numeric 2"=0.0, "Boolean 1"=FALSE, "Boolean 2"=FALSE, "Spin Program"=[], "Spin Prg v07"=[], "Time Stamp"=timestamp(0 s since 1904-01-01), "TabControl"=enum."Measure"}  # Device Queue
            n715 = Bundle By Name(cluster=w1535, "QueueAction"=DeviceQueue_Action."Arduino_Close") -> (w1533:T9)
          }
          frame True {
            w1538 = T9 {"QueueAction"=enum."TimeOut", "Numeric 1"=0.0, "Numeric 2"=0.0, "Boolean 1"=FALSE, "Boolean 2"=FALSE, "Spin Program"=[], "Spin Prg v07"=[], "Time Stamp"=timestamp(0 s since 1904-01-01), "TabControl"=enum."Measure"}  # Device Queue
            n716 = Bundle By Name(cluster=w1538, "QueueAction"=DeviceQueue_Action."Arduino_Init") -> (w1536:T9)
          }
        }
        n717 = Enqueue Element(queue=w1531, element=w1526, error in (no error)=w1529) -> (queue out=w1530:refnum<queue>, error out=w1528:errorcluster)  [unwired: 1 in, 1 out]
      }
      event "Program Spin Coater": Value Change {
        w1550 = T9 {"QueueAction"=enum."TimeOut", "Numeric 1"=0.0, "Numeric 2"=0.0, "Boolean 1"=FALSE, "Boolean 2"=FALSE, "Spin Program"=[], "Spin Prg v07"=[], "Time Stamp"=timestamp(0 s since 1904-01-01), "TabControl"=enum."Measure"}  # Device Queue
        n718 = event-data() -> ("NewVal"=w1539:T2)  [unwired: 1 in, 5 out]
        n719 = property on="Seconds to Spin" class="DigNum (strict)"() -> ("Value"=w1541:dbl[unit])  [unwired: 2 in, 2 out]
        n720 = node(w1541) -> (w1540:dbl)
        n721 = Bundle By Name(cluster=w1550, "QueueAction"=DeviceQueue_Action."Arduino_LoadProgram", "Spin Prg v07"=w1539, "Numeric 1"=w1540) -> (w1549:T9)
        n722 = Enqueue Element(queue=w1548, element=w1549, error in (no error)=w1546) -> (queue out=w1545:refnum<queue>, error out=w1544:errorcluster)  [unwired: 1 in, 1 out]
        n723 = property on="Measure_IntegrationTime" class="DigNum (strict)"() -> ("Value"=w1542:dbl[unit])  [unwired: 2 in, 2 out]
        n724 = property on="Measure_IntegrationTime" class="DigNum (strict)"("Val(Sgnl)"=w1542) -> ()  [unwired: 2 in, 2 out]
      }
      event "Measure_IntegrationTime", "SpectralStability_IntegrationTime": Value Change {
        w1563 = T9 {"QueueAction"=enum."TimeOut", "Numeric 1"=0.0, "Numeric 2"=0.0, "Boolean 1"=FALSE, "Boolean 2"=FALSE, "Spin Program"=[], "Spin Prg v07"=[], "Time Stamp"=timestamp(0 s since 1904-01-01), "TabControl"=enum."Measure"}  # Device Queue
        n725 = event-data() -> ("NewVal"=w1555:dbl[unit])  [unwired: 1 in, 5 out]
        n726 = property on="Calculate Frames" class="Bool (strict)"() -> ("Value"=w1551:bool)  [unwired: 2 in, 2 out]
        n727 = node(w1555) -> (w1554:dbl)
        n728 = property on="Tab Control" class="TabCtl (strict)"() -> ("Value"=w1553:T1)  [unwired: 2 in, 2 out]
        n729 = property on="Tab Control" class="TabCtl (strict)"() -> ("Value"=w1552:T1)  [unwired: 2 in, 2 out]
        n730 = case shown="\"Measure\"" w1553 {
          tunnel: w1563 -> [w1564 w1570 w1576]
          tunnel: [w1564 w1567 w1573] -> w1562
          tunnel: DeviceQueue_Action."Spectrometer_SetIntegrationTime" ("QueueAction") -> [_ w1569 w1575]
          tunnel: w1554 -> [_ w1568 w1574]
          tunnel: w1552 -> [_ w1566 w1571]
          tunnel: w1551 -> [_ w1565 _]
          frame Default {
          }
          frame "Measure" {
            n731 = Bundle By Name(cluster=w1570, "QueueAction"=w1569, "Numeric 1"=w1568, "Boolean 1"=w1565, "TabControl"=w1566) -> (w1567:T9)
          }
          frame "Spectral Stability" {
            n732 = Bundle By Name(cluster=w1576, "QueueAction"=w1575, "Numeric 1"=w1574, "Boolean 1"=FALSE, "TabControl"=w1571) -> (w1573:T9)
          }
        }
        n733 = Enqueue Element(queue=w1560, element=w1562, error in (no error)=w1559) -> (queue out=w1558:refnum<queue>, error out=w1557:errorcluster)  [unwired: 1 in, 1 out]
      }
      event "Frames": Value Change {
        w1584 = T9 {"QueueAction"=enum."TimeOut", "Numeric 1"=0.0, "Numeric 2"=0.0, "Boolean 1"=FALSE, "Boolean 2"=FALSE, "Spin Program"=[], "Spin Prg v07"=[], "Time Stamp"=timestamp(0 s since 1904-01-01), "TabControl"=enum."Measure"}  # Device Queue
        n734 = event-data() -> ()  [unwired: 1 in, 6 out]
        n735 = Bundle By Name(cluster=w1584, "QueueAction"=DeviceQueue_Action."Spectrometer_SetFrames", "Numeric 1"="Frames") -> (w1583:T9)
        n736 = Enqueue Element(queue=w1582, element=w1583, error in (no error)=w1580) -> (queue out=w1581:refnum<queue>, error out=w1579:errorcluster)  [unwired: 1 in, 1 out]
      }
      event "Seconds to Spin", "Seconds after Spin": Value Change {
        n737 = event-data() -> ()  [unwired: 1 in, 6 out]
        n738 = property on="Program Spin Coater" class="Arr (strict)"() -> ("Value"=w1586:T2)  [unwired: 2 in, 2 out]
        n739 = property on="Program Spin Coater" class="Arr (strict)"("Val(Sgnl)"=w1586) -> ()  [unwired: 2 in, 2 out]
      }
      event "Calculate Frames": Value Change {
        n740 = event-data() -> ("NewVal"=w1596:bool)  [unwired: 1 in, 5 out]
        n741 = case shown="False" w1596 {
          tunnel: [0 2] -> w1591
          tunnel: w1593 -> [w1598 w1607]
          tunnel: [w1598 w1605] -> w1594
          tunnel: w1592 -> [w1597 w1604]
          tunnel: [w1597 w1600] -> w1590
          frame False {
          }
          frame True {
            w1606 = T9 {"QueueAction"=enum."TimeOut", "Numeric 1"=0.0, "Numeric 2"=0.0, "Boolean 1"=FALSE, "Boolean 2"=FALSE, "Spin Program"=[], "Spin Prg v07"=[], "Time Stamp"=timestamp(0 s since 1904-01-01), "TabControl"=enum."Measure"}  # Device Queue
            n742 = property on="Measure_IntegrationTime" class="DigNum (strict)"() -> ("Value"=w1602:dbl[unit])  [unwired: 2 in, 2 out]
            n743 = node(w1602) -> (w1601:dbl)
            n744 = Bundle By Name(cluster=w1606, "QueueAction"=DeviceQueue_Action."Spectrometer_SetIntegrationTime", "Numeric 1"=w1601) -> (w1608:T9)
            n745 = Enqueue Element(queue=w1607, element=w1608, error in (no error)=w1604) -> (queue out=w1605:refnum<queue>, error out=w1600:errorcluster)  [unwired: 1 in, 1 out]
          }
        }
        n746 = property on="Frames" class="DigNum (strict)"("DisabledEnum"=w1591) -> ()  [unwired: 2 in, 2 out]
      }
      event "Record RefSpec": Value Change {
        w1617 = T9 {"QueueAction"=enum."TimeOut", "Numeric 1"=0.0, "Numeric 2"=0.0, "Boolean 1"=FALSE, "Boolean 2"=FALSE, "Spin Program"=[], "Spin Prg v07"=[], "Time Stamp"=timestamp(0 s since 1904-01-01), "TabControl"=enum."Measure"}  # Device Queue
        n747 = event-data() -> ()  [unwired: 1 in, 6 out]
        n748 = Bundle By Name(cluster=w1617, "QueueAction"=DeviceQueue_Action."Spectrometer_SetReference") -> (w1616:T9)
        n749 = Enqueue Element(queue=w1615, element=w1616, error in (no error)=w1612) -> (queue out=w1613:refnum<queue>, error out=w1611:errorcluster)  [unwired: 1 in, 1 out]
      }
      event "Measure_Preview", "SpectralStability_Preview": Value Change {
        n750 = event-data() -> ("NewVal"=w1618:bool)  [unwired: 1 in, 5 out]
        n751 = case shown="False" w1618 {
          tunnel: w1623 -> [w1625 w1630]
          tunnel: w1621 -> [w1624 w1629]
          tunnel: [w1625 w1628] -> w1620
          tunnel: [w1624 w1627] -> w1619
          frame False {
          }
          frame True {
            w1633 = T9 {"QueueAction"=enum."TimeOut", "Numeric 1"=0.0, "Numeric 2"=0.0, "Boolean 1"=FALSE, "Boolean 2"=FALSE, "Spin Program"=[], "Spin Prg v07"=[], "Time Stamp"=timestamp(0 s since 1904-01-01), "TabControl"=enum."Measure"}  # Device Queue
            n752 = property on="Tab Control" class="TabCtl (strict)"() -> ("Value"=w1626:T1)  [unwired: 2 in, 2 out]
            n753 = Bundle By Name(cluster=w1633, "QueueAction"=DeviceQueue_Action."Spectrometer_Preview", "TabControl"=w1626) -> (w1632:T9)
            n754 = Enqueue Element(queue=w1630, element=w1632, error in (no error)=w1629) -> (queue out=w1628:refnum<queue>, error out=w1627:errorcluster)  [unwired: 1 in, 1 out]
          }
        }
      }
      event "Measure:\nRecord_Darkspec", "SpectralStability:\nRecord_Darkspec": Value Change {
        w1641 = T9 {"QueueAction"=enum."TimeOut", "Numeric 1"=0.0, "Numeric 2"=0.0, "Boolean 1"=FALSE, "Boolean 2"=FALSE, "Spin Program"=[], "Spin Prg v07"=[], "Time Stamp"=timestamp(0 s since 1904-01-01), "TabControl"=enum."Measure"}  # Device Queue
        n755 = event-data() -> ()  [unwired: 1 in, 6 out]
        n756 = Bundle By Name(cluster=w1641, "QueueAction"=DeviceQueue_Action."Spectrometer_SetDarkspec") -> (w1640:T9)
        n757 = Enqueue Element(queue=w1639, element=w1640, error in (no error)=w1636) -> (queue out=w1637:refnum<queue>, error out=w1635:errorcluster)  [unwired: 1 in, 1 out]
      }
      event "StartMeasurement_Button": Value Change {
        w1648 = T6 {"QueueAction"=enum."TimeOut", "Data"=[], "Data_Raw"=[], "Data_Dark"=[], "Data_Ref"=[], "Device Information"=[], "Numeric Control"=0.0, "Boolean"=FALSE, "Wavelength"=[], "Time"=[], "Time Stamp"=timestamp(0 s since 1904-01-01), "Numeric Control 2"=0.0, "TabControl"=enum."Measure"}  # DataQueue
        w1656 = T9 {"QueueAction"=enum."TimeOut", "Numeric 1"=0.0, "Numeric 2"=0.0, "Boolean 1"=FALSE, "Boolean 2"=FALSE, "Spin Program"=[], "Spin Prg v07"=[], "Time Stamp"=timestamp(0 s since 1904-01-01), "TabControl"=enum."Measure"}  # Device Queue
        n758 = event-data() -> ()  [unwired: 1 in, 6 out]
        n759 = property on="Measure_Preview" class="Bool (strict)"("Value"=FALSE ("Preview")) -> ()  [unwired: 2 in, 2 out]
        n760 = Get Date/Time In Seconds() -> (seconds since 1Jan1904=w1642:timestamp)
        n761 = Bundle By Name(cluster=w1656, "QueueAction"=DeviceQueue_Action."Measure_InSituAdvanced", "Time Stamp"=w1642) -> (w1655:T9)
        n762 = Enqueue Element(queue=w1654, element=w1655, error in (no error)=w1652) -> (queue out=w1653:refnum<queue>, error out=w1643:errorcluster)  [unwired: 1 in, 1 out]
        n763 = Bundle By Name(cluster=w1648, "QueueAction"=DataQueue_Action."Measure_InSituSpinCoating", "Time Stamp"=w1642) -> (w1649:T6)
        n764 = Enqueue Element(queue=w1646, element=w1649, error in (no error)=w1643) -> (queue out=w1645:refnum<queue>, error out=w1644:errorcluster)  [unwired: 1 in, 1 out]
      }
      event "StartSpin_Button": Value Change {
        w1664 = T9 {"QueueAction"=enum."TimeOut", "Numeric 1"=0.0, "Numeric 2"=0.0, "Boolean 1"=FALSE, "Boolean 2"=FALSE, "Spin Program"=[], "Spin Prg v07"=[], "Time Stamp"=timestamp(0 s since 1904-01-01), "TabControl"=enum."Measure"}  # Device Queue
        n765 = event-data() -> ()  [unwired: 1 in, 6 out]
        n766 = Bundle By Name(cluster=w1664, "QueueAction"=DeviceQueue_Action."Arduino_StartProgram") -> (w1663:T9)
        n767 = Enqueue Element(queue=w1662, element=w1663, error in (no error)=w1658) -> (queue out=w1660:refnum<queue>, error out=w1659:errorcluster)  [unwired: 1 in, 1 out]
      }
      event "Milliseconds": Value Change {
        w1673 = T9 {"QueueAction"=enum."TimeOut", "Numeric 1"=0.0, "Numeric 2"=0.0, "Boolean 1"=FALSE, "Boolean 2"=FALSE, "Spin Program"=[], "Spin Prg v07"=[], "Time Stamp"=timestamp(0 s since 1904-01-01), "TabControl"=enum."Measure"}  # Device Queue
        n768 = event-data() -> ()  [unwired: 1 in, 6 out]
        n769 = Bundle By Name(cluster=w1673, "QueueAction"=DeviceQueue_Action."Arduino_SetMillis", "Numeric 1"="Milliseconds") -> (w1669:T9)
        n770 = Enqueue Element(queue=w1672, element=w1669, error in (no error)=w1670) -> (queue out=w1668:refnum<queue>, error out=w1667:errorcluster)  [unwired: 1 in, 1 out]
      }
      event "Speed": Value Change {
        w1682 = T9 {"QueueAction"=enum."TimeOut", "Numeric 1"=0.0, "Numeric 2"=0.0, "Boolean 1"=FALSE, "Boolean 2"=FALSE, "Spin Program"=[], "Spin Prg v07"=[], "Time Stamp"=timestamp(0 s since 1904-01-01), "TabControl"=enum."Measure"}  # Device Queue
        n771 = event-data() -> ()  [unwired: 1 in, 6 out]
        n772 = Bundle By Name(cluster=w1682, "QueueAction"=DeviceQueue_Action."Arduino_SetSpeed", "Numeric 1"="Speed") -> (w1678:T9)
        n773 = Enqueue Element(queue=w1681, element=w1678, error in (no error)=w1679) -> (queue out=w1677:refnum<queue>, error out=w1676:errorcluster)  [unwired: 1 in, 1 out]
      }
      event "Debug": Value Change {
        n774 = event-data() -> ()  [unwired: 1 in, 6 out]
        n775 = Select(t=u8 0, s="Debug", f=u8 2) -> (s? t:f=w1683:u8)
        n776 = property on="Milliseconds" class="DigNum (strict)"("DisabledEnum"=w1683) -> ()  [unwired: 2 in, 2 out]
        n777 = property on="Speed" class="DigNum (strict)"("DisabledEnum"=w1683) -> ()  [unwired: 2 in, 2 out]
      }
      event "Measure_FramesSpectrometer", "SpectralStability_FramesSpectrometer": Value Change {
        w1697 = T9 {"QueueAction"=enum."TimeOut", "Numeric 1"=0.0, "Numeric 2"=0.0, "Boolean 1"=FALSE, "Boolean 2"=FALSE, "Spin Program"=[], "Spin Prg v07"=[], "Time Stamp"=timestamp(0 s since 1904-01-01), "TabControl"=enum."Measure"}  # Device Queue
        n778 = event-data() -> ("NewVal"=w1691:dbl)  [unwired: 1 in, 5 out]
        n779 = property on="Tab Control" class="TabCtl (strict)"() -> ("Value"=w1690:T1)  [unwired: 2 in, 2 out]
        n780 = Bundle By Name(cluster=w1697, "QueueAction"=DeviceQueue_Action."Spectrometer_SetFrames", "Numeric 1"=w1691, "TabControl"=w1690) -> (w1698:T9)
        n781 = Enqueue Element(queue=w1695, element=w1698) -> (queue out=w1692:refnum<queue>)  [unwired: 2 in, 2 out]
      }
      event "Measure_MeasureSpectrum", "SpectralStability_MeasureSpectrum": Value Change {
        w1705 = T6 {"QueueAction"=enum."TimeOut", "Data"=[], "Data_Raw"=[], "Data_Dark"=[], "Data_Ref"=[], "Device Information"=[], "Numeric Control"=0.0, "Boolean"=FALSE, "Wavelength"=[], "Time"=[], "Time Stamp"=timestamp(0 s since 1904-01-01), "Numeric Control 2"=0.0, "TabControl"=enum."Measure"}  # DataQueue
        w1710 = T9 {"QueueAction"=enum."TimeOut", "Numeric 1"=0.0, "Numeric 2"=0.0, "Boolean 1"=FALSE, "Boolean 2"=FALSE, "Spin Program"=[], "Spin Prg v07"=[], "Time Stamp"=timestamp(0 s since 1904-01-01), "TabControl"=enum."Measure"}  # Device Queue
        n782 = event-data() -> ()  [unwired: 1 in, 6 out]
        n783 = property on="Tab Control" class="TabCtl (strict)"() -> ("Value"=w1699:T1)  [unwired: 2 in, 2 out]
        n784 = Get Date/Time In Seconds() -> (seconds since 1Jan1904=w1700:timestamp)
        n785 = Bundle By Name(cluster=w1710, "QueueAction"=DeviceQueue_Action."Measure_Spectrum", "Time Stamp"=w1700, "TabControl"=w1699) -> (w1711:T9)
        n786 = Enqueue Element(queue=w1708, element=w1711) -> (queue out=w1706:refnum<queue>)  [unwired: 2 in, 2 out]
        n787 = Bundle By Name(cluster=w1705, "QueueAction"=DataQueue_Action."Measure_Spectrum", "TabControl"=w1699) -> (w1702:T6)
        n788 = Enqueue Element(queue=w1703, element=w1702) -> (queue out=w1701:refnum<queue>)  [unwired: 2 in, 2 out]
      }
      event "SpectralStability_Record": Value Change {
        w1720 = T6 {"QueueAction"=enum."TimeOut", "Data"=[], "Data_Raw"=[], "Data_Dark"=[], "Data_Ref"=[], "Device Information"=[], "Numeric Control"=0.0, "Boolean"=FALSE, "Wavelength"=[], "Time"=[], "Time Stamp"=timestamp(0 s since 1904-01-01), "Numeric Control 2"=0.0, "TabControl"=enum."Measure"}  # DataQueue
        w1725 = T9 {"QueueAction"=enum."TimeOut", "Numeric 1"=0.0, "Numeric 2"=0.0, "Boolean 1"=FALSE, "Boolean 2"=FALSE, "Spin Program"=[], "Spin Prg v07"=[], "Time Stamp"=timestamp(0 s since 1904-01-01), "TabControl"=enum."Measure"}  # Device Queue
        n789 = event-data() -> ()  [unwired: 1 in, 6 out]
        n790 = property on="Duration/\nTimes" class="Bool (strict)"() -> ("Value"=w1713:bool)  [unwired: 2 in, 2 out]
        n791 = case shown="False" w1713 {
          tunnel: ["SpectralStability_\nMeasurementNumber" w1728] -> w1712
          frame False {
            # "Number"
          }
          frame True {
            # "Duration"
            n792 = property on="SpectralStability_\nPeriodicTime" class="DigNum (strict)"() -> ("Value"=w1730:dbl[unit])  [unwired: 2 in, 2 out]
            n793 = Divide(x="SpectralStability_Duration", y=w1730) -> (x/y=w1731:dbl)
            n794 = Round Toward +Infinity(x=w1731) -> (ceil(x): smallest int >= x=w1729:dbl)
            n795 = Increment(x=w1729) -> (x+1=w1728:dbl)
          }
        }
        n796 = Get Date/Time In Seconds() -> (seconds since 1Jan1904=w1714:timestamp)
        n797 = property on="Tab Control" class="TabCtl (strict)"() -> ("Value"=w1715:T1)  [unwired: 2 in, 2 out]
        n798 = Bundle By Name(cluster=w1725, "QueueAction"=DeviceQueue_Action."Measure_SpectralStability", "Time Stamp"=w1714, "TabControl"=w1715, "Numeric 1"=w1712) -> (w1726:T9)
        n799 = property on="SS_StepsLeft" class="DigNum (strict)"("Value"=w1712) -> ()  [unwired: 2 in, 2 out]
        n800 = Enqueue Element(queue=w1723, element=w1726) -> (queue out=w1721:refnum<queue>)  [unwired: 2 in, 2 out]
        n801 = Bundle By Name(cluster=w1720, "QueueAction"=DataQueue_Action."Measure_SpectralStability", "TabControl"=w1715, "Time Stamp"=w1714, "Numeric Control"=w1712) -> (w1717:T6)
        n802 = Enqueue Element(queue=w1718, element=w1717) -> (queue out=w1716:refnum<queue>)  [unwired: 2 in, 2 out]
      }
      event "Automatically \nadjust count": Value Change {
        n803 = event-data() -> ("NewVal"=w1739:bool)  [unwired: 1 in, 5 out]
        n804 = Select(t=u8 2, s=w1739, f=u8 0) -> (s? t:f=w1733:u8)
        n805 = property on="Spectra Count" class="DigNum (strict)"("DisabledEnum"=w1733) -> ()  [unwired: 2 in, 2 out]
      }
      event "Duration/Times": Value Change {
        n806 = event-data() -> ("NewVal"=w1745:bool)  [unwired: 1 in, 5 out]
        n807 = case shown="False" w1745 {
          tunnel: [FALSE TRUE] -> w1744
          tunnel: [TRUE FALSE] -> w1743
          frame False {
          }
          frame True {
          }
        }
        n808 = property on="SpectralStability_Duration" class="DigNum (strict)"("Visible"=w1744) -> ()  [unwired: 2 in, 2 out]
        n809 = property on="SpectralStability_\nMeasurementNumber" class="DigNum (strict)"("Visible"=w1743) -> ()  [unwired: 2 in, 2 out]
      }
      event "Tab Control": Value Change {
        w1750 = FALSE ("SpectralStability_Preview")
        n810 = event-data() -> ("NewVal"=w1753:T1)  [unwired: 1 in]
        n811 = case shown="\"Spectral Stability\"" w1753 {
          tunnel: w1755 -> [w1758 w1771 w1786]
          tunnel: [w1758 w1760 w1777] -> w1752
          tunnel: w1754 -> [w1757 w1770 w1785]
          tunnel: w1753 -> [_ w1769 w1784]
          tunnel: [w1757 w1759 w1776] -> w1751
          frame Default {
          }
          frame "Measure" {
            w1773 = T9 {"QueueAction"=enum."TimeOut", "Numeric 1"=0.0, "Numeric 2"=0.0, "Boolean 1"=FALSE, "Boolean 2"=FALSE, "Spin Program"=[], "Spin Prg v07"=[], "Time Stamp"=timestamp(0 s since 1904-01-01), "TabControl"=enum."Measure"}  # Device Queue
            n812 = property on="Measure_IntegrationTime" class="DigNum (strict)"() -> ("Value"=w1768:dbl[unit])  [unwired: 2 in, 2 out]
            n813 = node(w1768) -> (w1767:dbl)
            n814 = Bundle By Name(cluster=w1773, "QueueAction"=DeviceQueue_Action."Spectrometer_SetIntegrationTime", "Numeric 1"=w1767, "TabControl"=w1769) -> (w1764:T9)
            n815 = property on="Measure_FramesSpectrometer" class="DigNum (strict)"() -> ("Value"=w1762:dbl)  [unwired: 2 in, 2 out]
            n816 = Enqueue Element(queue=w1771, element=w1764, error in (no error)=w1770) -> (queue out=w1766:refnum<queue>, error out=w1765:errorcluster)  [unwired: 1 in, 1 out]
            n817 = Bundle By Name(cluster=w1764, "QueueAction"=DeviceQueue_Action."Spectrometer_SetFrames", "Numeric 1"=w1762) -> (w1761:T9)
            n818 = Enqueue Element(queue=w1766, element=w1761, error in (no error)=w1765) -> (queue out=w1760:refnum<queue>, error out=w1759:errorcluster)  [unwired: 1 in, 1 out]
          }
          frame "Spectral Stability" {
            w1788 = T9 {"QueueAction"=enum."TimeOut", "Numeric 1"=0.0, "Numeric 2"=0.0, "Boolean 1"=FALSE, "Boolean 2"=FALSE, "Spin Program"=[], "Spin Prg v07"=[], "Time Stamp"=timestamp(0 s since 1904-01-01), "TabControl"=enum."Measure"}  # Device Queue
            n819 = property on="SpectralStability_IntegrationTime" class="DigNum (strict)"() -> ("Value"=w1775:dbl[unit])  [unwired: 2 in, 2 out]
            n820 = node(w1775) -> (w1783:dbl)
            n821 = property on="SpectralStability_FramesSpectrometer" class="DigNum (strict)"() -> ("Value"=w1774:dbl)  [unwired: 2 in, 2 out]
            n822 = Bundle By Name(cluster=w1788, "QueueAction"=DeviceQueue_Action."Spectrometer_SetIntegrationTime", "Numeric 1"=w1783, "TabControl"=w1784) -> (w1780:T9)
            n823 = Enqueue Element(queue=w1786, element=w1780, error in (no error)=w1785) -> (queue out=w1782:refnum<queue>, error out=w1781:errorcluster)  [unwired: 1 in, 1 out]
            n824 = Bundle By Name(cluster=w1780, "QueueAction"=DeviceQueue_Action."Spectrometer_SetFrames", "Numeric 1"=w1774) -> (w1778:T9)
            n825 = Enqueue Element(queue=w1782, element=w1778, error in (no error)=w1781) -> (queue out=w1777:refnum<queue>, error out=w1776:errorcluster)  [unwired: 1 in, 1 out]
          }
        }
        n826 = property on="SpectralStability_Preview" class="Bool (strict)"("Value"=w1750) -> ()  [unwired: 2 in, 2 out]
        n827 = property on="Measure_Preview" class="Bool (strict)"("Value"=w1750) -> ()  [unwired: 2 in, 2 out]
      }
    }
  }
  n828 = disable-structure shown="Disabled" {
    frame Disabled {
      w1790 = T9 {"QueueAction"=enum."TimeOut", "Numeric 1"=0.0, "Numeric 2"=0.0, "Boolean 1"=FALSE, "Boolean 2"=FALSE, "Spin Program"=[], "Spin Prg v07"=[], "Time Stamp"=timestamp(0 s since 1904-01-01), "TabControl"=enum."Measure"}  # Device Queue
      w1793 = T9 {"QueueAction"=enum."TimeOut", "Numeric 1"=0.0, "Numeric 2"=0.0, "Boolean 1"=FALSE, "Boolean 2"=FALSE, "Spin Program"=[], "Spin Prg v07"=[], "Time Stamp"=timestamp(0 s since 1904-01-01), "TabControl"=enum."Measure"}  # Device Queue
      n829 = Bundle By Name(cluster=w1790, "QueueAction"=DeviceQueue_Action."Arduino_SetSpeed") -> (w1791:T9)  [unwired: 1 in]
      n830 = Bundle By Name(cluster=w1793, "QueueAction"=DeviceQueue_Action."Arduino_SetSpeed") -> (w1792:T9)  [unwired: 1 in]
      n831 = Enqueue Element(element=w1791) -> ()  [unwired: 3 in, 3 out]
      n832 = Enqueue Element(element=w1792) -> ()  [unwired: 3 in, 3 out]
    }
    frame Enabled {
    }
  }
  n833 = Release Queue(queue=w9) -> ()  [unwired: 2 in, 3 out]
  n834 = Release Queue(queue=w10) -> ()  [unwired: 2 in, 3 out]
